vi "UHR-Fleezers Control (fpga) - Lorentz 1.vi"() -> ()   [LabVIEW 2014]
doc: "UHR-Fleezers Instrument Control Code (fpga)"
uses:
  <vilib>/Platform/TimedLoop/XDataNode/timing_clust.ctl
  <vilib>/Platform/TimedLoop/XDataNode/nitl_modes.ctl
  <vilib>/Platform/TimedLoop/XDataNode/wakeup.ctl
  <vilib>/rvi/Emulation/niFpgaGetClockAttributes.vi
  <vilib>/rvi/Emulation/niFpgaSctlEmulationGetInTimedLoop.vi
  <vilib>/rvi/Emulation/niFpgaEmulationReportErrorSimple.vi
  <vilib>/rvi/Emulation/niFpgaProcessEmulError.vi
  <vilib>/rvi/eio/common/nirviEmuTemplateMethod_errors.vi
  <vilib>/rvi/interface/RandomDataEmulation/niFpgaRandomDataHandleErrors.vi
  <vilib>/rvi/Emulation/niFpgaCriticalErrorInLSC.vi
  <vilib>/eio/EIONode/EIONode.xnode
  <vilib>/eio/EIOMethodNode/EIOMethodNode.xnode
  <vilib>/rvi/DataTransferAndStorage/Container/XNode/niFpgaContainer.xnode
  <vilib>/rvi/interface/RandomDataEmulation/nirviRandomDataFpgaReadWriteTemplate.vi
  <vilib>/addons/control/pid/fpga.llb/XNode/niFpgaPID.xnode
  <vilib>/Platform/TimedLoop/XDataNode/XDataNode.xnode
  <vilib>/Platform/TimedLoop/XDataNode/XDNodeRunTimeDep.lvlib
panel:
  in  "Tab Control":T1(tab)=enum."MCL trap control"
  in  "Set 3":bool
  in  "Set 2":bool=TRUE
  in  "Set 1":bool=TRUE
  in  "Trap Pos to FIFO":bool
  in  "N of AI1 Int Acq Sets":i16=2 min=1 max=3 step=1
  out "AI Late Counter":u8
  in  "ai count":u16=400
  in  "+ phase":bool
  in  "Phase count adjustment":i16
  out "Relative phase":i16
  in  "AI to FIFO":bool
  out "BD1 Frequency Out 1":u64
  out "BD1 Frequency Out 2":u64
  out "Trap Pos FIFO Timeout":u16
  out "Trap AI FIFO Timeout":u16
  in  "Trap FIFO Set Timeout":i32
  in  "Tab Control 2":T2(tab)
  in  "FB output range":cluster{"output low":i16, "output high":i16}={"output low"=0, "output high"=3000}
  in  "FB Gains":T3={"proportional gain (Kc)"=10, "integral gain (Kc*Ts/Ti)"=5, "derivative gain (Kc*Td/Ts)"=0}
  in  "RD":bool
  in  "Swap F1 and F2":bool
  in  "Cont. Scan":bool
  in  "Abort scan":bool
  in  "Cycles per step":u64
  in  "Scan BD":bool
  in  "Number of scans":u16
  in  "Scan steps":u64
  in  "Scan freq.  increment":i64
  out "Scanning":bool
  in  "Start scan":bool
  in  "OSK Bd 1":bool
  in  "Reset Bd 1":bool
  in  "PMODE":bool
  in  "Direct RF Box \nCommunication":bool
  in  "Data BD 2":u8 format="%08b"
  in  "Data BD 1":u8 format="%08b"
  in  "Address":u8 format="%02x"
  in  "Update Data":bool
  in  "FPGA Controls\n RF Box":bool
  in  "Number Interlace Cycles":u8=2 min=1 max=3
  in  "Interlace Off Parameters":u8=1 min=1 max=3
  in  "Interlace ON/OFF":bool
  out "DIO Relative phase":i16
  in  "Phase count adjustment (DIO)":i16
  in  "+ phase (DIO)":bool
  out "DIO Late Counter":u8
  in  "DIO count 1 (ticks)":u16=400
  in  "DIO count 2 (ticks)":u16=400
  in  "DIO count 3 (ticks)":u16=400
  out "AI2 Y Sum Set 2":i16
  out "AI2 Y Sum Set 1":i16
  in  "FB Setpoint Set 1":i16 min=0 step=1
  in  "FB Reset Set 1":bool
  in  "FB On/Off Set 1":bool
  in  "FB Reset Set 2":bool
  in  "FB On/Off Set 2":bool
  in  "FB Setpoint Set 2":i16 min=0 step=1
  out "Scan I":u64
  in  "Amp switch delay":u8=5
  in  "BD 2 Amplitude 1":u16
  in  "BD 1 Amplitude 1":u16
  in  "BD 2 Frequency 1":u64
  in  "BD 1 Frequency 1":u64
  in  "BD 2 Amplitude 2":u16
  in  "BD 1 Amplitude 2":u16
  in  "BD 2 Frequency 2":u64
  in  "BD 1 Frequency 2":u64
  in  "BD 2 Amplitude 3":u16
  in  "BD 1 Amplitude 3":u16
  in  "BD 2 Frequency 3":u64
  in  "BD 1 Frequency 3":u64
  in  "BD 1 Delay (ticks)":u8
  in  "BD 2 Delay (Ticks)":u8 caption="Count(Ticks)"
  in  "Next trap write delay (ticks)":u8 caption="Count(Ticks)"
  out "Piezo X out":u16
  out "Piezo Y out":u16
  in  "Piezo Trap ON/Off (AO3)":u16
  in  "Piezo Trap X (AO5)":u16
  in  "Piezo Trap Y (AO4)":u16
  in  "Trap pos. FB Range":T4={"FB2 output low"=-1.0, "FB2 output high"=0.999969482421875}
  in  "FB Min frequency":u64
  in  "FB Max Frequency":u64
  in  "Dynamic Force FB (Ronen)":bool
  in  "Negate Diff?":bool
  in  "Diff FB Measurement?":bool
  in  "FB Trig Integrate":u32=1
  out "TTrig?":bool
  in  "TTrig Negate Pos":bool=TRUE
  out "Trap Pos FB Int Signal":fxp<+/-,24,9> format="%.18g"
  out "Trap Pos FB Int-Norm Signal":fxp<+/-,16,1> format="%.16g"
  in  "FPGA TTrig Thresh":i64
  in  "FPGA Trap Trig":bool
  out "Trap Pos FB Action":i64
  in  "Trap Pos. FB Offset Factor":i64
  in  "Trap Pos. FB Mult Factor":i64=2
  in  "Trap Pos. FB Reset":bool
  in  "Trap Pos FB Monitor T1 or T2":bool
  in  "AI1 X Scale":u16
  in  "Trap Pos FB Int Count":u16=100
  in  "Trap Pos FB Negate Action":bool
  out "AI1 X Set 2":fxp<+/-,16,1>
  out "AI1 X Set 1":fxp<+/-,16,1>
  in  "Trap Pos. FB SP":fxp<+/-,16,1>
  in  "Force feedback":bool
  out "TTrig Sig":i64
  out "TTrig Fin Thresh":i64
  in  "B factor":fxp<+/-,32,16>
  in  "Trap Pos. FB Gains":T5={"proportional gain (Kc)"=0.999969482421875, "integral gain (Kc*Ts/Ti)"=0.999969482421875, "derivative gain (Kc*Td/Ts)"=0.0}
  in  "1D or 2D Scan?":bool
  in  "Abort scan (MCL)":bool
  in  "MCL Scan Axis":bool
  in  "Cont. Scan (MCL)":bool
  out "Scan I (MCL)":u64
  in  "Number of scans (MCL)":u16
  out "Scanning MCL":bool
  in  "Scan steps (MCL)":u64
  in  "Cycles per step (MCL)":u64
  in  "Scan freq.  increment (MCL)":i16
  in  "Start scan (MCL)":bool
  in  "AO2":i16
  in  "AO1":i16
  out "MCL Late Counter":u8
  in  "MCL count":u32=800
  out "MCL Relative Phase":i16
  in  "Phase count adjustment (MCL)":i16
  in  "+ phase (MCL)":bool
  out "APD2 int gate":bool
  out "APD3 out state":bool
  in  "APD Gate Operating Mode":u8 max=2 step=1
  in  "Invert APD Gate":bool
  in  "APD Gate OFF Count":u16=100
  in  "APD Gate ON Count":u16=300
  out "APD 1 Gate Late Counter":u8
  out "APD 1 Gate Relative Phase":i16
  in  "Phase count adjustment (APD 1 Gate)":i16
  in  "+ phase (APD 1 Gate)":bool
  out "APD 2 Counts 0":u32
  out "APD 2 Counts 1":u32
  out "APD 1 Counts 0":u32
  out "APD 1 Counts 1":u32
  out "APD1 out state":bool
  in  "APD AO scale factor":i16=1
  in  "APD to FIFO":bool
  in  "APD Acq Rate Count":u32=20000000
  out "APD Acq Late Counter":u8
  out "APD Acq Relative Phase":i16
  in  "Phase Count Adjustment (APD Acq)":i16
  in  "+ phase (APD Acq)":bool
  in  "Phase count adjustment (APD 2 Gate)":i16
  out "APD 2 Gate Late Counter":u8
  out "APD 2 Gate Relative Phase":i16
  in  "+ phase (APD 2 Gate)":bool
  out "APD2 out state":bool
  out "APD 3 Counts 0":u32
  out "APD 3 Counts 1":u32
  out "APD 3 Gate Late Counter":u8
  in  "Phase count adjustment (APD 3 Gate)":i16
  out "APD 3 Gate Relative Phase":i16
  in  "+ phase (APD 3 Gate)":bool
  out "APD1 int gate":bool
  out "APD3 int gate":bool
  in  "D3":i16
  in  "I3":i16=5
  in  "P3":i16=10
  in  "Green Filter Flipper":bool
  in  "Green FB Count":u16=1200
  out "Green Late Counter":u8
  out "Green FB Relative Phase":i16
  in  "Phase count adjustment (Green FB)":i16=10
  in  "+ phase (Green FB)":bool
  out "Green FB Sum":i16
  in  "Green int current ON count adj":u16=150
  in  "Current Out":u16=30000
  in  "Green FB On/Off":bool
  in  "Green FB Setpoint":i16=250 min=0 step=1
  in  "Green FB Reset":bool
  in  "Operating Mode 2":u8=2 max=2 step=1
  in  "Invert GI 2":bool
  in  "Green interlace OFF count 2":u16=900
  in  "Green interlace ON count 2":u16=300
  out "GI Late Counter 2":u8
  out "GI Relative phase 2":i16
  in  "Phase count adjustment (GI) 2":i16=20
  in  "+ phase (GI) 2":bool
  in  "Green interlace OFF count":u16=100
  out "GI Relative phase":i16
  in  "Phase count adjustment (GI)":i16
  in  "+ phase (GI)":bool
  in  "Green interlace ON count":u16=300
  out "GI Late Counter":u8
  in  "Invert GI":bool
  in  "Operating Mode":u8 max=2 step=1
  in  "+ phase (RI)":bool
  out "RI Relative phase":i16
  out "RI Late Counter":u8
  in  "Red interlace ON count":u16=300
  in  "Red interlace OFF count":u16=100
  in  "Invert RI":bool
  in  "Red Laser Operating Mode":u8 max=2 step=1
  in  "Phase count adjustment (RI)":i16
  out "Red FB Intensity":i16
  in  "RI Current Out":u16=30000
  in  "Red FB On/Off":bool
  in  "D4":i16
  in  "I4":i16=5
  in  "P4":i16=10
  in  "Red FB Setpoint":i16=250 min=0 step=1
  in  "Red FB Reset":bool
  in  "RI Operating Mode 2":u8=2 max=2 step=1
  in  "Invert RI 2":bool
  in  "Phase count adjustment (BI AO)":i16=20
  in  "Blue current ON count adj (AO)":u16=150
  in  "BI Current Out":i16=30000
  in  "Blue FB On/Off":bool
  in  "D5":i16
  in  "I5":i16=5
  in  "P5":i16=10
  in  "Blue FB Setpoint":i16=250 min=0 step=1
  in  "Blue FB Reset":bool
  in  "BI Operating Mode (AO)":u8=2 max=2 step=1
  in  "Invert BI (AO)":bool
  in  "Blue OFF count (AO)":u16=900
  in  "Blue ON count (AO)":u16=300
  out "BI Late Counter (AO)":u8
  out "BI Relative phase (AO)":i16
  in  "+ phase (BI AO)":bool
  in  "Phase count adjustment (BI D)":i16
  in  "Blue Laser Operating Mode (D)":u8 max=2 step=1
  in  "Invert BI (D)":bool
  in  "Blue interlace OFF count (D)":u16=100
  in  "Blue interlace ON count (D)":u16=300
  out "Blue Late Counter (D)":u8
  out "BI Relative phase (D)":i16
  in  "+ phase (BI D)":bool
  out "Blue Intensity":i16
  # "Only one of these can be on\nat a time:"
  # "Raster Scan AOD"
  # "1 (X)"
  # "2 (Y)"
  # "IR Intensity Feedback (RF BD 1)"
  # "False is usual, True is external loop method"
  # "Parameters if using the external RF switching loop"
  # "Parameters if using the usual internal RF switching method"
  # "FB Triggering Excitation Laser"
  # "Trap Pos. FB Gains"
  # "Trap Pos. FB Range"
  # "AO1 (Y)"
  # "2D"
  # "1D"
  # "AO2 (X)"
  # "APD AO for aligning"
  # "Detection Loop"
  # "Green fluorescent laser digital gate interlacing loop"
  # "0 Forced ON\n1 Forced OFF\n2 Interlacing"
  # "Green FB Gains"
  # "Red fluorescent laser digital gate interlacing loop"
  # "Detection Loop"
  # "0 Forced ON\n1 Forced OFF\n2 Interlacing"
  # "Analog/FB Control Loop\n(Disabled)"
  # "Digital Control Loop"
  # "Blue laser intensity reading"
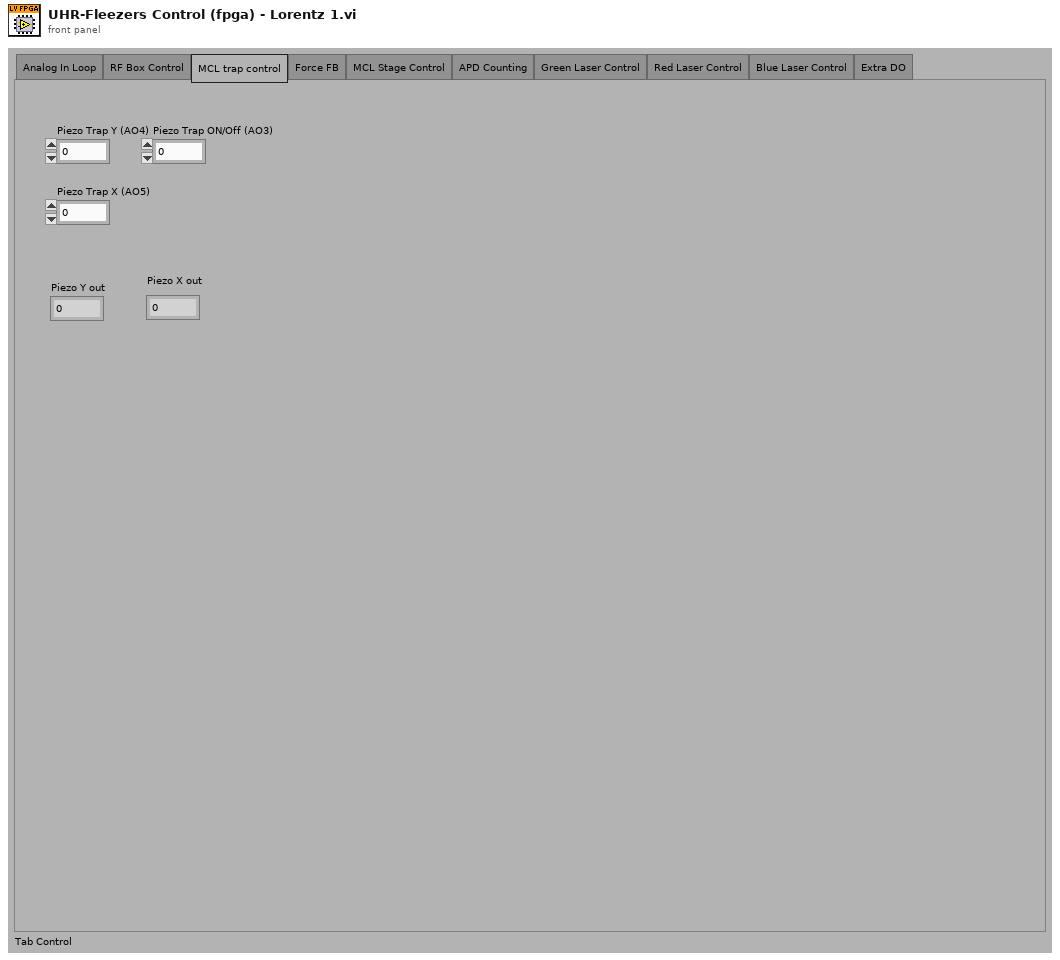
[diagram p1: front panel]
types:
  T1 = enum32{"Analog In Loop", "RF Box Control", "MCL trap control", "Force FB", "MCL Stage Control", "APD Counting", "Green Laser Control", "Red Laser Control", "Blue Laser Control", "Extra DO"}
  T2 = enum32{"Controls", "Interlacing Frequency and Amplitude Values", "Oscillate trap from memory"}
  T3 = cluster{"proportional gain (Kc)":i16, "integral gain (Kc*Ts/Ti)":i16, "derivative gain (Kc*Td/Ts)":i16}
  T4 = cluster{"FB2 output low":fxp<+/-,16,1>, "FB2 output high":fxp<+/-,16,1>}
  T5 = cluster{"proportional gain (Kc)":fxp<+/-,16,1>, "integral gain (Kc*Ts/Ti)":fxp<+/-,16,1>, "derivative gain (Kc*Td/Ts)":fxp<+/-,16,1>}
  T6 = typedef "XDNodeRunTimeDep.lvlib/timing_clust.ctl" = cluster{"Expected End [f-1]":u64, "Actual End [f-1]":u64, "Finished Late? [f-1]":bool, "Expected End [i-1]":u64, "Actual End [i-1]":u64, "Finished Late? [i-1]":bool, "Expected Start [i]":u64, "Actual Start [i]":u64, "Expected Start [f]":u64, "Actual Start [f]":u64, "Source Name":string, "Structure Name":string, "Period":i64, "Deadline":i64, "Offset":i64, "Start":i64, "Priority":i32, "Timeout":i32, "Mode":T7, "Wakeup Reason":T8, "Error":errorcluster, "Source Type":string, "Secondary Source Type":string, "Global End Time":u64, "Global Start Time":u64, "Frame Duration":u64, "Iteration Duration":u64, "Assigned CPU":i32, "I/O Scan Engine Mode":u32}
  T7 = typedef "XDNodeRunTimeDep.lvlib/nitl_modes.ctl" = enum32{"No Change", "Process missed periods, maintain original phase", "Discard missed periods, maintain original phase", "Process missed periods, ignore original phase", "Discard missed periods, ignore original phase"}
  T8 = typedef "XDNodeRunTimeDep.lvlib/wakeup.ctl" = enum32{"Normal", "Aborted", "Asynchronous wakeup", "Timing source error", "Timed loop error", "Timeout"}
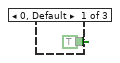
[diagram p2: hidden frame]
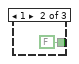
[diagram p3: hidden frame]
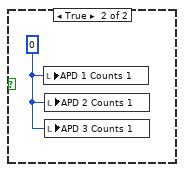
[diagram p5: hidden frame]
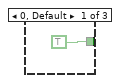
[diagram p7: hidden frame]
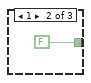
[diagram p8: hidden frame]
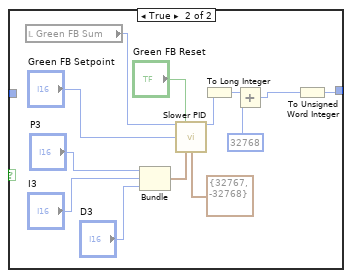
[diagram p11: hidden frame]
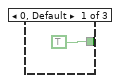
[diagram p12: hidden frame]
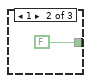
[diagram p13: hidden frame]
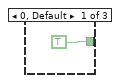
[diagram p14: hidden frame]
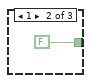
[diagram p15: hidden frame]
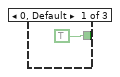
[diagram p17: hidden frame]
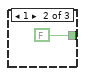
[diagram p18: hidden frame]
diagram:
  w1 = i16 0
  w7 = FALSE
  w5 = FALSE
  # "Control of MCL trap"
  # "timing array current index"
  # "timing array"
  # "timing counter (phase adjusted here)"
  # "late counter"
  n1 = flat-sequence "FPGA initialization to do before running any of the loops" {
    tunnel: [u16 0 ("DIO count 3 (ticks)")] -> w3
    tunnel: [w15] -> _
    frame #0 {
      w14 = FALSE ("Enable")
      # "BD 2 (Y)"
      # "BD 1 (X)"
      # "Start up expansion chassis early\nto avoid delays later"
      # "This pin controls udclk on the RF boards.\nWhen initially configuring the boards, this pin needs to be\nconfigured as a high impedance input.  Later it will be switched\nto an output."
      # "Initial setting of DIO data and \naddress to low (before reset).  \nThis needs to happen before the other\ncontrol method loops execute."
      n2 = xnode "FPGA I/O Node"("Chassis2/Mod1/AO0"=u16 0 ("Chassis2/Mod4/AO0")) -> ("Chassis2/Mod2/AI0"=w15:i16)  [unwired: 2 in, 2 out]
      n3 = xnode "FPGA I/O Method Node"("Enable"=w14) -> ()  [unwired: 1 in, 1 out]
      n4 = xnode "FPGA I/O Method Node"("Enable"=w14) -> ()  [unwired: 1 in, 1 out]
      n5 = xnode "FPGA I/O Node"("Connector1/DIO0"=FALSE, "Connector1/DIO1"=FALSE, "Connector1/DIO2"=FALSE, "Connector1/DIO3"=FALSE, "Connector1/DIO4"=FALSE, "Connector1/DIO5"=FALSE, "Connector1/DIO6"=FALSE, "Connector1/DIO7"=FALSE, "Connector1/DIO8"=FALSE, "Connector1/DIO9"=FALSE, "Connector1/DIO10"=FALSE, "Connector1/DIO11"=FALSE, "Connector1/DIO12"=FALSE, "Connector1/DIO13"=FALSE, "Connector1/DIO15"=FALSE, "Connector1/DIO20"=FALSE, "Connector1/DIO21"=FALSE, "Connector1/DIO22"=FALSE, "Connector1/DIO23"=FALSE, "Connector1/DIO24"=FALSE, "Connector1/DIO25"=FALSE, "Connector1/DIO26"=FALSE, "Connector1/DIO27"=FALSE, "Connector1/DIO14"=FALSE) -> ()  [unwired: 24 in, 24 out]
    }
  }
  n6 = local read "AO1"() -> (w12:i16)
  n7 = local read "AO2"() -> (w11:i16)
  n8 = node-c288() -> (w10:T6)  [unwired: 1 in]
  n9 = To Unsigned Long Integer(number=w3) -> (unsigned 32bit integer=w8:u32)
  n10 = timed-loop "RF box board DIO control: control bits" {
    timing: w10 -> [_]
    timing-out: [_] -> w9
    tunnel: [w44] -> _
    tunnel: w3 -> [w44]
    stop <- FALSE stop-if-true
    n11 = xnode "FPGA I/O Node"("Connector1/DIO16"="RD", "Connector1/DIO17"="PMODE", "Connector1/DIO18"="OSK Bd 1", "Connector1/DIO19"="Reset Bd 1", "Connector0/DIO3"="Green Filter Flipper") -> ()  [unwired: 5 in, 5 out]
  }
  n12 = while "RF box board DIO control: parallel communication" {
    shift-right: [w65] -> _
    shift-left: w3 -> [w64]
    shift-right: [w63] -> _
    shift-left: FALSE ("Swap F1 and F2") -> [w62]
    shift-right: [w57] -> _
    shift-left: u64 0 -> [w58]
    shift-right: [w54] -> _
    shift-left: i16 0 -> [w55]
    shift-right: [w53] -> _
    shift-left: w1 -> [w56]
    shift-right: [w52] -> _
    shift-left: w1 -> [w51]
    stop <- FALSE stop-if-true
    n13 = flat-sequence {
      tunnel: w62 -> [w69]
      tunnel: w64 -> [w67]
      tunnel: [w69] -> w61
      tunnel: [w68] -> w60
      tunnel: [w67] -> w59
      tunnel: [w83] -> w65
      tunnel: [w82] -> w63
      tunnel: w61 -> [w81]
      tunnel: w60 -> [w79]
      tunnel: w59 -> [w78]
      tunnel: w58 -> [w77]
      tunnel: [w76] -> w57
      tunnel: w56 -> [w75]
      tunnel: w55 -> [w74]
      tunnel: [w73] -> w54
      tunnel: [w72] -> w53
      tunnel: [w71] -> w52
      tunnel: w51 -> [w70]
      frame #0 {
        n14 = call "Loop Timer"("Count(Ticks)"=w67) -> ("Tick Count(Ticks)"=w68:u16)
      }
      frame #1 {
        n15 = flat-sequence {
          tunnel: ["FPGA Controls\n RF Box"] -> w80
          tunnel: w81 -> [w87]
          tunnel: w75 -> [w86]
          tunnel: w74 -> [w85]
          tunnel: w70 -> [w84]
          tunnel: [w148] -> w83
          tunnel: [w161] -> w82
          tunnel: w80 -> [w160]
          tunnel: w79 -> [w154]
          tunnel: w78 -> [w151]
          tunnel: w77 -> [w126]
          tunnel: [w125] -> w76
          tunnel: ["Piezo Trap Y (AO4)"] -> w73
          tunnel: ["Piezo Trap X (AO5)"] -> w72
          tunnel: ["Piezo Trap ON/Off (AO3)"] -> w71
          frame #0 {
            n16 = case shown="True" "FPGA Controls\n RF Box" {
              tunnel: w87 -> [_ w92]
              tunnel: w86 -> [_ w91]
              tunnel: w85 -> [_ w90]
              tunnel: w84 -> [_ w89]
              frame False {
              }
              frame True {
                n17 = flat-sequence {
                  tunnel: w92 -> [w102]
                  tunnel: w91 -> [w119]
                  tunnel: w90 -> [w118]
                  tunnel: w89 -> [w117]
                  frame #0 {
                    n18 = First Call?() -> (First Call?: T/F=w93:bool)
                    n19 = case shown="True" w93 {
                      frame False {
                      }
                      frame True {
                        # "BD 2"
                        # "BD 1"
                        # "If first time data updated, be sure to set WR high and UDCLK low\nbefore setting data and address bits."
                        n20 = xnode "FPGA I/O Method Node"("Enable"=TRUE) -> ("FPGA I/O Out"=w95:refnum<k21>)  [unwired: 1 in]
                        n21 = xnode "FPGA I/O Method Node"("Enable"=TRUE) -> ("FPGA I/O Out"=w98:refnum<k21>)  [unwired: 1 in]
                        n22 = xnode "FPGA I/O Node"("Connector1/DIO15"=TRUE) -> ()  [unwired: 1 in, 1 out]
                        n23 = xnode "FPGA I/O Node"("I/O Item"=FALSE ("Connector1/DIO30"), "FPGA I/O In"=w95) -> ()  [unwired: 1 out]
                        n24 = xnode "FPGA I/O Node"("I/O Item"=FALSE ("Connector1/DIO30"), "FPGA I/O In"=w98) -> ()  [unwired: 1 out]
                      }
                    }
                  }
                  frame #1 {
                    n25 = case shown="False" FALSE {
                      tunnel: w102 -> [w104 _]
                      frame False {
                        # "Usual operation"
                        n26 = disable-structure shown="Disabled" {
                          disable-tunnel: w104 -> [w106 _]
                          disable-tunnel: "Amp switch delay" -> [w105 _]
                          frame Disabled {
                            n27 = flat-sequence "BD 2 (Y)" {
                              tunnel: w106 -> [w108]
                              tunnel: w105 -> [w109]
                              frame #0 {
                                n28 = call "Wait7"("Count(Ticks)"="BD 2 Delay (Ticks)") -> ()  [unwired: 1 out]
                              }
                              frame #1 {
                                # "switch frequency"
                                n29 = xnode "FPGA I/O Node"("Connector1/DIO37"=w108) -> ()  [unwired: 1 in, 1 out]
                              }
                              frame #2 {
                                # "~5 ticks is usual"
                                n30 = call "Wait5"("Count(Ticks)"=w109) -> ()  [unwired: 1 out]
                              }
                              frame #3 {
                                # "this switches amplitude"
                                # "switch amplitude"
                                # "send udclk high"
                                n31 = xnode "FPGA I/O Node"("Connector1/DIO29"=TRUE ("Connector1/DIO15")) -> ()  [unwired: 1 in, 1 out]
                              }
                              frame #4 {
                                # "reset to be ready for next\ncycle"
                                # "send udclk low"
                                n32 = xnode "FPGA I/O Node"("Connector1/DIO29"=FALSE ("Connector1/DIO15")) -> ()  [unwired: 1 in, 1 out]
                              }
                            }
                          }
                          frame Enabled {
                          }
                        }
                        n33 = flat-sequence "BD 1 (X)" {
                          tunnel: w104 -> [w113]
                          tunnel: "Amp switch delay" -> [w114]
                          frame #0 {
                            n34 = call "Wait6"("Count(Ticks)"="BD 1 Delay (ticks)") -> ()  [unwired: 1 out]
                          }
                          frame #1 {
                            # "switch frequency"
                            n35 = xnode "FPGA I/O Node"("Connector1/DIO36"=w113) -> ()  [unwired: 1 in, 1 out]
                          }
                          frame #2 {
                            # "~5 ticks is usual"
                            n36 = call "Wait4"("Count(Ticks)"=w114) -> ()  [unwired: 1 out]
                          }
                          frame #3 {
                            # "this switches amplitude"
                            # "switch amplitude"
                            # "send udclk high"
                            n37 = xnode "FPGA I/O Node"("Connector1/DIO30"=TRUE ("Connector1/DIO15")) -> ()  [unwired: 1 in, 1 out]
                          }
                          frame #4 {
                            # "reset to be ready for next\ncycle"
                            # "send udclk low"
                            n38 = xnode "FPGA I/O Node"("Connector1/DIO30"=FALSE ("Connector1/DIO15")) -> ()  [unwired: 1 in, 1 out]
                          }
                        }
                      }
                      frame True {
                        # "Operation when you need a long delay for either X or Y to synchonize AOD light out phase (> ~100 ticks)."
                        # "Trigger the external loop by sending the boolean FSK value through a FIFO"
                      }
                    }
                  }
                  frame #2 {
                    n39 = xnode "FPGA I/O Node"("Connector0/AO4"=w118, "Connector0/AO5"=w119, "Connector0/AO3"=w117) -> ()  [unwired: 3 in, 3 out]
                  }
                }
              }
            }
          }
          frame #1 {
            # "This is the prior cycle's on time"
            # "increment timing\nindex, reset to 0 if \nend of matrix"
            # "Reset to begginning (1) when number of cycles reached."
            # "timing index"
            # "build byte stacks for writing data\n(must correspond to addresses array constant)"
            # "Timing housekeeping"
            # "Adjust phase if late\n(maintains constant phase relationship between cycles)"
            n40 = feedback #1(u8 0 ("t")) -> (w157:u8)
            n41 = Increment(x=w157) -> (x+1=w200:u8)
            n42 = Increment(x="Number Interlace Cycles") -> (x+1=w195:u8)
            n43 = Equal?(x=w200, y=w195) -> (x = y?=w202:bool)
            n44 = Select(t=u8 1, s=w202, f=w200) -> (s? t:f=w156:u8)
            n45 = feedback-in #1(w156) -> ()
            n46 = Increment(x=w156) -> (x+1=w197:u8)
            n47 = Equal?(x=w197, y=w195) -> (x = y?=w198:bool)
            n48 = Select(t=u8 1, s=w198, f=w197) -> (s? t:f=w194:u8)
            n49 = Select(t=w194, s="Interlace ON/OFF", f="Interlace Off Parameters") -> (s? t:f=w127:u8)
            n50 = case shown="1, Default" w127 {
              tunnel: [w246 w455 "BD 1 Frequency 3"] -> w190
              tunnel: [w289 "BD 2 Frequency 2" "BD 2 Frequency 3"] -> w179
              tunnel: ["BD 2 Amplitude 1" "BD 2 Amplitude 2" "BD 2 Amplitude 3"] -> w136
              tunnel: [w255 w453 "BD 1 Amplitude 3"] -> w139
              tunnel: "FB output range" -> [w259 w450 _]
              tunnel: w126 -> [w254 w452 w468]
              tunnel: [w246 w452 w468] -> w125
              tunnel: "FB Gains" -> [w241 w451 _]
              frame 1, Default {
                w273 = fxp<+/-,24,9> 0.0 ("AI1 X Set 2")
                w267 = u16 0
                w285 = u64 0 ("f")
                # "Added by Ronen -\nUpper and Lower \nLimits for the FB \ngenerated frequency\nto avoid losing bead \nwhen tether breaks"
                # "Changed by Ronen - correction \nby PID is now implemented not on \nthe Base BD1 frequency but on the last\nfrequency sent."
                # "BD1 Amp 1"
                # "This signal integration happens no matter what\nso that correct setpoints can be chosen before \nturning on the FB."
                # "Trap 1"
                n51 = local read "AI1 X Set 2"() -> (w249:fxp<+/-,16,1>)
                n52 = local read "AI1 X Set 1"() -> (w270:fxp<+/-,16,1>)
                n53 = local read "Scanning"() -> (w290:bool)
                n54 = Multiply(x=w249, y="B factor") -> (x*y=w247:fxp<+/-,48,17>)
                n55 = Or(x=w290, y="Start scan") -> (x .or. y?=w283:bool)
                n56 = case shown="True" "Diff FB Measurement?" {
                  tunnel: w247 -> [w308 w317]
                  tunnel: w270 -> [w307 w318]
                  tunnel: [w305 w309] -> w271
                  frame False {
                    n57 = Select(t=w307, s="Trap Pos FB Monitor T1 or T2", f=w308) -> (s? t:f=w305:fxp<+/-,48,17>)
                  }
                  frame True {
                    n58 = Subtract(x=w318, y=w317) -> (x-y=w310:fxp<+/-,48,17>)
                    n59 = Not(x="Negate Diff?") -> (.not. x?=w316:bool)
                    n60 = Boolean To (0,1)(Boolean="Negate Diff?") -> (0, 1=w314:i16)
                    n61 = Boolean To (0,1)(Boolean=w316) -> (0, 1=w315:i16)
                    n62 = Negate(x=w314) -> (-x=w313:i16)
                    n63 = Add(x=w313, y=w315) -> (x+y=w311:i16)
                    n64 = Multiply(x=w311, y=w310) -> (x*y=w309:fxp<+/-,63,32>)
                  }
                }
                n65 = Not(x="Abort scan") -> (.not. x?=w281:bool)
                n66 = And(x=w281, y=w283) -> (x .and. y?=w280:bool)
                n67 = case "For raster scanning" shown="True" w280 {
                  tunnel: [u64 0 w440] -> w286
                  tunnel: "Start scan" -> [_ w425]
                  frame False {
                    n68 = local write "Scanning"(FALSE ("scanning")) -> ()
                  }
                  frame True {
                    w409 = i64 0
                    w408 = u64 0
                    # "scan incr."
                    # "freq. incr. mult."
                    # "count steps"
                    # "count number of cycles"
                    n69 = feedback #2(w408) -> (w437:u64)
                    n70 = Select(t=w408, s=w425, f=w437) -> (s? t:f=w439:u64)
                    n71 = Increment(x=w439) -> (x+1=w436:u64)
                    n72 = Greater?(x="Cycles per step", y=w436) -> (0:w418:bool)
                    n73 = Select(t=w436, s=w418, f=w408) -> (s? t:f=w435:u64)
                    n74 = feedback-in #2(w435) -> ()
                    n75 = feedback #3(w408) -> (w434:u64)
                    n76 = Select(t=w408, s=w425, f=w434) -> (s? t:f=w429:u64)
                    n77 = Increment(x=w429) -> (x+1=w433:u64)
                    n78 = Add(x="Scan steps", y="Scan steps") -> (x+y=w432:u64)
                    n79 = Select(t=w429, s=w418, f=w433) -> (s? t:f=w413:u64)
                    n80 = Greater?(x=w432, y=w413) -> (0:w412:bool)
                    n81 = Select(t=w413, s=w412, f=w408) -> (s? t:f=w430:u64)
                    n82 = feedback-in #3(w430) -> ()
                    n83 = Equal?(x="Scan steps", y=w413) -> (x = y?=w417:bool)
                    n84 = Greater?(x="Scan steps", y=w429) -> (0:w428:bool)
                    n85 = feedback #4(w409) -> (w431:i64)
                    n86 = Select(t=w409, s=w425, f=w431) -> (s? t:f=w415:i64)
                    n87 = Increment(x=w415) -> (x+1=w427:i64)
                    n88 = Decrement(x=w415) -> (x-1=w426:i64)
                    n89 = Select(t=w427, s=w428, f=w426) -> (s? t:f=w416:i64)
                    n90 = Select(t=w415, s=w417, f=w416) -> (s? t:f=w414:i64)
                    n91 = Select(t=w415, s=w418, f=w414) -> (s? t:f=w410:i64)
                    n92 = Select(t=w410, s=w412, f=w409) -> (s? t:f=w411:i64)
                    n93 = feedback-in #4(w411) -> ()
                    n94 = feedback #5(w408) -> (w424:u64)
                    n95 = Select(t=w408, s=w425, f=w424) -> (s? t:f=w420:u64)
                    n96 = Increment(x=w420) -> (x+1=w421:u64)
                    n97 = Select(t=w420, s=w412, f=w421) -> (s? t:f=w419:u64)
                    n98 = Greater?(x="Number of scans", y=w419) -> (0:w405:bool)
                    n99 = Multiply(x="Scan freq.  increment", y=w415) -> (x*y=w440:i64)
                    n100 = Select(t=TRUE, s="Cont. Scan", f=w405) -> (s? t:f=w404:bool)
                    "Scanning" <- w404
                    n101 = Select(t=w419, s=w404, f=w408) -> (s? t:f=w422:u64)
                    n102 = feedback-in #5(w422) -> ()
                    n103 = Increment(x=w419) -> (x+1=→"Scan I":u64)
                  }
                }
                n104 = feedback #6(w267) -> (w266:u16)
                n105 = Increment(x=w266) -> (x+1=w268:u16)
                n106 = Greater Or Equal?(x=w268, y="Trap Pos FB Int Count") -> (x >= y?=w253:bool)
                n107 = Select(t=w267, s=w253, f=w268) -> (s? t:f=w269:u16)
                n108 = feedback-in #6(w269) -> ()
                n109 = feedback #7(w273) -> (w272:fxp<+/-,24,9>)
                n110 = Add(x=w271, y=w272) -> (x+y=w265:fxp<+/-,24,9>)
                n111 = case "For intensity feedback" shown="True" "FB On/Off Set 1" {
                  tunnel: [w442 w448] -> w255
                  tunnel: w259 -> [_ w449]
                  tunnel: "BD 1 Amplitude 1" -> [w442 _]
                  tunnel: w241 -> [_ w443]
                  frame False {
                  }
                  frame True {
                    n112 = local read "AI2 Y Sum Set 1"() -> (w446:i16)
                    n113 = call "Slower PID.vi"("process variable"=w446, "reset?"="FB Reset Set 1", "setpoint"="FB Setpoint Set 1", "PID gains (x 2^8)"=w443, "output range"=w449) -> ("output"=w444:i16)  [unwired: 10 out]
                    n114 = To Unsigned Word Integer(number=w444) -> (unsigned 16bit integer=w448:u16)
                  }
                }
                n115 = Select(t=w273, s=w253, f=w265) -> (s? t:f=w276:fxp<+/-,24,9>)
                n116 = feedback-in #7(w276) -> ()
                n117 = Divide(x=w265, y="Trap Pos FB Int Count") -> (x/y=w260:fxp<+/-,16,1>)
                n118 = feedback #8(fxp<+/-,24,9> 0.0 ("AI1 X Set 2")) -> (w277:fxp<+/-,24,9>)
                n119 = Select(t=w265, s=w253, f=w277) -> (s? t:f=w278:fxp<+/-,24,9>)
                "Trap Pos FB Int Signal" <- w278
                n120 = feedback-in #8(w278) -> ()
                n121 = feedback #9(fxp<+/-,16,1> 0.0 ("Trap Pos FB Int-Norm Signal")) -> (w262:fxp<+/-,16,1>)
                n122 = Select(t=w260, s=w253, f=w262) -> (s? t:f=w261:fxp<+/-,16,1>)
                "Trap Pos FB Int-Norm Signal" <- w261
                n123 = feedback-in #9(w261) -> ()
                n124 = case "For position feedback" shown="True" "Force feedback" {
                  tunnel: [i64 0 w324] -> w258
                  tunnel: w260 -> [_ w321]
                  tunnel: w253 -> [_ w320]
                  frame False {
                  }
                  frame True {
                    n125 = feedback #10(i64 0) -> (w323:i64)
                    n126 = case shown="True" w320 {
                      tunnel: [w325 w329] -> w324
                      tunnel: w323 -> [w325 _]
                      tunnel: w321 -> [_ w328]
                      frame False {
                      }
                      frame True {
                        n127 = xnode ("PID")("process variable"=w328, "reset?"="Trap Pos. FB Reset", "setpoint"="Trap Pos. FB SP", "PID gains"="Trap Pos. FB Gains", "output range"="Trap pos. FB Range") -> ("output"=w338:fxp<+/-,16,1>)
                        n128 = Negate(x=w338) -> (-x=w337:fxp<+/-,17,2>)
                        n129 = Select(t=w337, s="Trap Pos FB Negate Action", f=w338) -> (s? t:f=w334:fxp<+/-,17,2>)
                        n130 = Scale By Power Of 2(n=u32 15, x=u32 1) -> (x*2^n=w331:u32)
                        n131 = Multiply(x=w334, y=w331) -> (x*y=w330:fxp<+/-,17,17>)
                        n132 = To Quad Integer(1:w330) -> (0:w342:i64)
                        "Trap Pos FB Action" <- w342
                        n133 = Multiply(x=w342, y="Trap Pos. FB Mult Factor") -> (x*y=w340:i64)
                        n134 = Add(x=w340, y="Trap Pos. FB Offset Factor") -> (x+y=w329:i64)
                        n135 = disable-structure shown="Disabled" {
                          disable-tunnel: w329 -> [w349 _]
                          frame Disabled {
                            w353 = u32 0
                            n136 = feedback #11() -> (w350:i64)  [unwired: 1 in]
                            n137 = Add(x=w349, y=w350) -> (x+y=w347:i64)
                            n138 = feedback #12(w353) -> (w355:u32)
                            n139 = Increment(x=w355) -> (x+1=w344:u32)
                            n140 = Greater Or Equal?(x=w344, y="FB Trig Integrate") -> (x >= y?=w345:bool)
                            n141 = Select(t=i64 0, s=w345, f=w347) -> (s? t:f=w351:i64)
                            n142 = feedback-in #11(w351) -> ()
                            n143 = Select(t=w353, s=w345, f=w344) -> (s? t:f=w354:u32)
                            n144 = feedback-in #12(w354) -> ()
                            n145 = And(x=w345, y="FPGA Trap Trig") -> (x .and. y?=w352:bool)
                            n146 = case "Trap FB trigger excitation laser ON" shown="True" w352 {
                              tunnel: w347 -> [_ w359]
                              tunnel: w344 -> [_ w357]
                              frame False {
                              }
                              frame True {
                                n147 = Not(x="TTrig Negate Pos") -> (.not. x?=w366:bool)
                                n148 = Boolean To (0,1)(Boolean="TTrig Negate Pos") -> (0, 1=w364:i16)
                                n149 = Boolean To (0,1)(Boolean=w366) -> (0, 1=w365:i16)
                                n150 = Negate(x=w364) -> (-x=w363:i16)
                                n151 = Add(x=w363, y=w365) -> (x+y=w362:i16)
                                n152 = Multiply(x=w362, y=w359) -> (x*y=w361:i64)
                                "TTrig Sig" <- w361
                                n153 = Multiply(x="FPGA TTrig Thresh", y=w357) -> (x*y=w358:i64)
                                "TTrig Fin Thresh" <- w358
                                n154 = Greater Or Equal?(x=w361, y=w358) -> (x >= y?=w360:bool)
                                n155 = case shown="True" w360 {
                                frame False {
                                }
                                frame True {
                                w369 = TRUE ("Green FB On/Off")
                                w371 = u8 2 ("Operating Mode")
                                n156 = local write "Operating Mode 2"(w371) -> ()
                                n157 = local write "Operating Mode"(w371) -> ()
                                n158 = local write "Green FB On/Off"(w369) -> ()
                                n159 = local write "FPGA Trap Trig"(FALSE ("FPGA Trap Trig")) -> ()
                                "TTrig?" <- w369
                                }
                                }
                              }
                            }
                          }
                          frame Enabled {
                          }
                        }
                      }
                    }
                    n160 = feedback-in #10(w324) -> ()
                  }
                }
                n161 = And(x="Force feedback", y="Dynamic Force FB (Ronen)") -> (x .and. y?=w243:bool)
                n162 = case shown="True" w243 {
                  tunnel: w258 -> [w296 w300]
                  tunnel: [w295 w299] -> w256
                  tunnel: w254 -> [_ w298]
                  tunnel: w253 -> [_ w297]
                  frame False {
                    # "(BD1 Frequency 1)"
                    n163 = Add(x="BD 1 Frequency 1", y=w296) -> (x+y=w295:u64)
                  }
                  frame True {
                    n164 = case shown="True" w297 {
                      tunnel: w300 -> [_ w304]
                      tunnel: [w301 w303] -> w299
                      tunnel: w298 -> [w301 w302]
                      frame False {
                      }
                      frame True {
                        n165 = Add(x=w302, y=w304) -> (x+y=w303:u64)
                      }
                    }
                  }
                }
                n166 = Select(t=w285, s="Scan BD", f=w286) -> (s? t:f=w284:u64)
                n167 = Select(t=w286, s="Scan BD", f=w285) -> (s? t:f=w287:u64)
                n168 = Add(x=w284, y="BD 2 Frequency 1") -> (x+y=w289:u64)
                n169 = Compound Arithmetic op=ADD(i64 0 ("f"), w256, w287) -> (w252:u64)
                n170 = In Range and Coerce(upper limit="FB Max Frequency", x=w252, lower limit="FB Min frequency") -> (coerced(x)=w246:u64)  [unwired: 1 out]
                "BD1 Frequency Out 1" <- w246
              }
              frame 2 {
                # "Trap 2"
                n171 = case shown="True" "FB On/Off Set 2" {
                  tunnel: ["BD 1 Amplitude 2" w463] -> w453
                  tunnel: w450 -> [_ w464]
                  tunnel: w451 -> [_ w461]
                  frame False {
                  }
                  frame True {
                    n172 = local read "AI2 Y Sum Set 2"() -> (w466:i16)
                    n173 = call "Slower PID.vi"("process variable"=w466, "reset?"="FB Reset Set 2", "setpoint"="FB Setpoint Set 2", "PID gains (x 2^8)"=w461, "output range"=w464) -> ("output"=w462:i16)  [unwired: 10 out]
                    n174 = To Unsigned Word Integer(number=w462) -> (unsigned 16bit integer=w463:u16)
                  }
                }
                n175 = Add(x="BD 1 Frequency 2", y=i64 0 ("f")) -> (x+y=w455:u64)
                "BD1 Frequency Out 2" <- w455
              }
              frame 3 {
                # "Fluorescence period"
              }
            }
            n176 = feedback-in #13(w154) -> ()
            n177 = feedback #13(w154) -> (w153:u16)
            n178 = Select(t=w156, s="Interlace ON/OFF", f="Interlace Off Parameters") -> (s? t:f=w193:u8)
            n179 = Subtract(x=w154, y=w153) -> (x-y=w152:u16)
            n180 = Subtract "The error"(x=w152, y=w151) -> (x-y=w129:u16)
            n181 = case shown="1, Default" w193 {
              tunnel: ["DIO count 1 (ticks)" "DIO count 2 (ticks)" "DIO count 3 (ticks)"] -> w150
              frame 1, Default {
              }
              frame 2 {
              }
              frame 3 {
              }
            }
            n182 = Number To Boolean Array(number=w129) -> (Boolean array=w130:bool[])
            n183 = Or Array Elements(Boolean array=w130) -> (logical OR=w128:bool)
            n184 = Boolean To (0,1)(Boolean=w128) -> (0, 1=w135:i16)
            n185 = To Unsigned Byte Integer(number=w135) -> (unsigned 8bit integer=w132:u8)
            n186 = feedback #14(u8 0) -> (w133:u8)
            n187 = Add(x=w132, y=w133) -> (x+y=w131:u8)
            "DIO Late Counter" <- w131
            n188 = feedback-in #14(w131) -> ()
            n189 = Subtract(x=w150, y=w129) -> (x-y=w149:u16)
            n190 = Split Number(x=w190) -> (hi(x)=w189:u32, lo(x)=w188:u32)
            n191 = Split Number(x=w179) -> (hi(x)=w184:u32, lo(x)=w183:u32)
            n192 = Boolean To (0,1)(Boolean="+ phase (DIO)") -> (0, 1=w146:i16)
            n193 = Split Number(x=w189) -> (lo(x)=w187:u16)  [unwired: 1 out]
            n194 = Split Number(x=w188) -> (hi(x)=w186:u16, lo(x)=w185:u16)
            n195 = Split Number(x=w184) -> (lo(x)=w182:u16)  [unwired: 1 out]
            n196 = Split Number(x=w183) -> (hi(x)=w181:u16, lo(x)=w180:u16)
            n197 = Split Number(x=w139) -> (hi(x)=w141:u8, lo(x)=w140:u8)
            n198 = Split Number(x=w136) -> (hi(x)=w138:u8, lo(x)=w137:u8)
            n199 = Split Number(x=w187) -> (hi(x)=w178:u8, lo(x)=w177:u8)
            n200 = Split Number(x=w186) -> (hi(x)=w176:u8, lo(x)=w175:u8)
            n201 = Split Number(x=w182) -> (hi(x)=w171:u8, lo(x)=w170:u8)
            n202 = Split Number(x=w185) -> (hi(x)=w174:u8, lo(x)=w173:u8)
            n203 = Split Number(x=w181) -> (hi(x)=w169:u8, lo(x)=w168:u8)
            n204 = Split Number(x=w180) -> (hi(x)=w167:u8, lo(x)=w166:u8)
            n205 = Multiply(x=w146, y="Phase count adjustment (DIO)") -> (x*y=w142:i16)
            n206 = feedback #15(i16 0) -> (w144:i16)
            n207 = Subtract(x=w144, y=w142) -> (x-y=w143:i16)
            "DIO Relative phase" <- w143
            n208 = feedback-in #15(w143) -> ()
            n209 = Add(x=w149, y=w142) -> (x+y=w148:u16)
            n210 = Build Array "BD 1 A Stack"(w141, w140) -> (w163:u8[])
            n211 = Build Array "BD 2 A Stack"(w138, w137) -> (w162:u8[])
            n212 = Build Array "BD 1 nu Stack"(w178, w177, w176, w175, w174, w173) -> (w172:u8[])
            n213 = Build Array "BD 2 nu Stack"(w171, w170, w169, w168, w167, w166) -> (w165:u8[])
            n214 = case shown="2" w127 {
              tunnel: [w233 w236] -> w161
              tunnel: [u8 10 u8 4] -> w164
              tunnel: "Swap F1 and F2" -> [w234 w236]
              frame 2 {
                # "F2"
                n215 = Not(x=w234) -> (.not. x?=w233:bool)
              }
              frame 1, Default {
                # "low chooses F1"
                # "F1"
              }
            }
            n216 = case "If FPGA is controlling (toggling) RF synth" shown="True" w160 {
              tunnel: w172 -> [_ w209]
              tunnel: w165 -> [_ w208]
              tunnel: w164 -> [_ w207]
              tunnel: w163 -> [_ w206]
              tunnel: w162 -> [_ w205]
              frame False {
              }
              frame True {
                # "Write next amp.\n(wait until beginning of next loop iteration to update)"
                n217 = flat-sequence "Update the next F1 and F2 frequency value (the actual frequency won't change until FSK is switched).\nThen load the next amplitude value into buffer, but don't update it until the next cycle." {
                  tunnel: w208 -> [w211]
                  tunnel: w209 -> [w212]
                  tunnel: [w212] -> w204
                  tunnel: [w211] -> w203
                  tunnel: w207 -> [w213]
                  tunnel: w204 -> [w215]
                  tunnel: w203 -> [w214]
                  tunnel: w206 -> [w226]
                  tunnel: w205 -> [w225]
                  frame #0 {
                    # "To possibly send\nthese writes to very\nend of loop (for x and\ny phase adjust)"
                    n218 = call "Wait8"("Count(Ticks)"="Next trap write delay (ticks)") -> ()  [unwired: 1 out]
                  }
                  frame #1 {
                    n219 = for {
                      tunnel: w215 -> [w221] mode=indexing
                      tunnel: w214 -> [w220] mode=indexing
                      tunnel: w213 -> [w218]
                      i -> [w219]
                      # "Write next freq."
                      n220 = To Unsigned Byte Integer(number=w219) -> (unsigned 8bit integer=w216:u8)
                      n221 = Add(x=w218, y=w216) -> (x+y=w217:u8)
                      n222 = call "write to RF synth bd.vi"("Address Byte"=w217, "BD 2 Byte"=w220, "BD 1 Byte"=w221) -> ()
                    }
                  }
                  frame #2 {
                    w222 = TRUE ("Connector1/DIO15")
                    # "send udclk high\n(BD 1 and 2)"
                    n223 = xnode "FPGA I/O Node"("Connector1/DIO30"=w222, "Connector1/DIO29"=w222) -> ()  [unwired: 2 in, 2 out]
                  }
                  frame #3 {
                    w223 = FALSE ("Connector1/DIO15")
                    n224 = xnode "FPGA I/O Node"("Connector1/DIO30"=w223, "Connector1/DIO29"=w223) -> ()  [unwired: 2 in, 2 out]
                  }
                  frame #4 {
                    n225 = for {
                      tunnel: w226 -> [w232] mode=indexing
                      tunnel: w225 -> [w231] mode=indexing
                      tunnel: u8 33 -> [w229]
                      i -> [w230]
                      n226 = To Unsigned Byte Integer(number=w230) -> (unsigned 8bit integer=w227:u8)
                      n227 = Add(x=w229, y=w227) -> (x+y=w228:u8)
                      n228 = call "write to RF synth bd.vi"("Address Byte"=w228, "BD 2 Byte"=w231, "BD 1 Byte"=w232) -> ()
                    }
                  }
                }
              }
            }
            "Piezo Y out" <- "Piezo Trap Y (AO4)"
            "Piezo X out" <- "Piezo Trap X (AO5)"
          }
        }
      }
    }
  }
  n229 = disable-structure shown="Disabled" {
    disable-tunnel: w3 -> [w473 _]
    frame Disabled {
      n230 = while "Excitation laser intensity feedback measurement (all lasers)" {
        shift-right: [w474] -> _
        shift-left: w473 -> [w479]
        stop <- FALSE stop-if-true
        n231 = flat-sequence {
          tunnel: w479 -> [w481]
          tunnel: [w482] -> w477
          tunnel: [w481] -> w475
          tunnel: [w488] -> w478
          tunnel: w477 -> [w488]
          tunnel: [w487] -> w476
          tunnel: w475 -> [w487]
          tunnel: [w500] -> w474
          tunnel: w478 -> [w511]
          tunnel: w476 -> [w508]
          frame #0 {
            n232 = call "Loop Timer9"("Count(Ticks)"=w481) -> ("Tick Count(Ticks)"=w482:u16)
          }
          frame #1 {
            # "Design note:\n\nAll lasers need to be measured at the same \ntime because the AI expansion module\ncannot independently time the measurements\nwithin our requirements: their is dead time.\n\nThis probably wouldn't be an issue with the built\nin AI on the fpga board itself."
            n233 = xnode "FPGA I/O Node"("Connector1/DIO35"=TRUE) -> ("Chassis2/Mod2/AI2"=→"Blue Intensity":i16, "Chassis2/Mod2/AI1"=→"Red FB Intensity":i16, "Chassis2/Mod2/AI0"=→"Green FB Sum":i16)  [unwired: 4 in, 4 out]
          }
          frame #2 {
            n234 = feedback-in #16(w511) -> ()
            n235 = feedback #16(w511) -> (w510:u16)
            n236 = Subtract(x=w511, y=w510) -> (x-y=w509:u16)
            n237 = xnode "FPGA I/O Node"("Connector1/DIO35"=FALSE) -> ()  [unwired: 1 in, 1 out]
            n238 = Subtract(x=w509, y=w508) -> (x-y=w490:u16)
            n239 = Subtract(x="Green FB Count", y=w490) -> (x-y=w504:u16)
            n240 = Number To Boolean Array(number=w490) -> (Boolean array=w491:bool[])
            n241 = Or Array Elements(Boolean array=w491) -> (logical OR=w489:bool)
            n242 = Boolean To (0,1)(Boolean="+ phase (Green FB)") -> (0, 1=w502:i16)
            n243 = Boolean To (0,1)(Boolean=w489) -> (0, 1=w496:i16)
            n244 = Multiply(x=w502, y="Phase count adjustment (Green FB)") -> (x*y=w497:i16)
            n245 = Add(x=w504, y=w497) -> (x+y=w500:u16)
            n246 = To Unsigned Byte Integer(number=w496) -> (unsigned 8bit integer=w493:u8)
            n247 = feedback #17(i16 0) -> (w499:i16)
            n248 = Subtract(x=w499, y=w497) -> (x-y=w498:i16)
            "Green FB Relative Phase" <- w498
            n249 = feedback-in #17(w498) -> ()
            n250 = feedback #18(u8 0) -> (w494:u8)
            n251 = Add(x=w493, y=w494) -> (x+y=w492:u8)
            "Green Late Counter" <- w492
            n252 = feedback-in #18(w492) -> ()
          }
        }
      }
    }
    frame Enabled {
    }
  }
  n253 = while "RF box board direct communication loop" {
    tunnel: w3 -> [_]
    stop <- FALSE stop-if-true
    n254 = case "Whether to use direct communication method (only use one method at a time)" shown="True" "Direct RF Box \nCommunication" {
      frame False {
      }
      frame True {
        n255 = case shown="True" "Update Data" {
          frame False {
          }
          frame True {
            n256 = flat-sequence {
              frame #0 {
                n257 = First Call?() -> (First Call?: T/F=w515:bool)
                n258 = case shown="True" w515 {
                  frame False {
                  }
                  frame True {
                    # "If first time data updated, be sure to set WR high\nbefore setting data and address bits."
                    n259 = flat-sequence {
                      frame #0 {
                        n260 = xnode "FPGA I/O Node"("Connector1/DIO15"=TRUE) -> ()  [unwired: 1 in, 1 out]
                      }
                      frame #1 {
                        n261 = call "Wait"("Count(Ticks)"=u8 40 ("DO Delay 3 (Ticks)")) -> ()  [unwired: 1 out]
                      }
                    }
                  }
                }
              }
              frame #1 {
                n262 = Number To Boolean Array(number="Address") -> (Boolean array=w564:bool[])
                n263 = Number To Boolean Array(number="Data BD 1") -> (Boolean array=w565:bool[])
                n264 = Number To Boolean Array(number="Data BD 2") -> (Boolean array=w534:bool[])
                n265 = Index Array(array=w565, index=7) -> (element=w549:bool)
                n266 = Index Array(array=w565, index=6) -> (element=w548:bool)
                n267 = Index Array(array=w565, index=5) -> (element=w547:bool)
                n268 = Index Array(array=w565, index=4) -> (element=w546:bool)
                n269 = Index Array(array=w565, index=3) -> (element=w545:bool)
                n270 = Index Array(array=w565, index=2) -> (element=w544:bool)
                n271 = Index Array(array=w565, index=1) -> (element=w543:bool)
                n272 = Index Array(array=w565, index=0) -> (element=w542:bool)
                n273 = Index Array(array=w564, index=5) -> (element=w541:bool)
                n274 = Index Array(array=w564, index=4) -> (element=w540:bool)
                n275 = Index Array(array=w564, index=3) -> (element=w539:bool)
                n276 = Index Array(array=w564, index=2) -> (element=w538:bool)
                n277 = Index Array(array=w564, index=1) -> (element=w537:bool)
                n278 = Index Array(array=w564, index=0) -> (element=w536:bool)
                n279 = Index Array(array=w534, index=7) -> (element=w525:bool)
                n280 = Index Array(array=w534, index=6) -> (element=w524:bool)
                n281 = Index Array(array=w534, index=5) -> (element=w523:bool)
                n282 = Index Array(array=w534, index=4) -> (element=w522:bool)
                n283 = Index Array(array=w534, index=3) -> (element=w521:bool)
                n284 = Index Array(array=w534, index=2) -> (element=w520:bool)
                n285 = Index Array(array=w534, index=1) -> (element=w519:bool)
                n286 = Index Array(array=w534, index=0) -> (element=w518:bool)
                n287 = xnode "FPGA I/O Node"("Connector1/DIO0"=w549, "Connector1/DIO1"=w548, "Connector1/DIO2"=w547, "Connector1/DIO3"=w546, "Connector1/DIO4"=w545, "Connector1/DIO5"=w544, "Connector1/DIO6"=w543, "Connector1/DIO7"=w542, "Connector1/DIO8"=w541, "Connector1/DIO9"=w540, "Connector1/DIO10"=w539, "Connector1/DIO11"=w538, "Connector1/DIO12"=w537, "Connector1/DIO13"=w536, "Connector1/DIO20"=w525, "Connector1/DIO21"=w524, "Connector1/DIO22"=w523, "Connector1/DIO23"=w522, "Connector1/DIO24"=w521, "Connector1/DIO25"=w520, "Connector1/DIO26"=w519, "Connector1/DIO27"=w518) -> ()  [unwired: 22 in, 22 out]
              }
              frame #2 {
                # "wait and then apply write signal"
                n288 = call "Wait2"("Count(Ticks)"=u8 40 ("DO Delay 1 (Ticks)")) -> ()  [unwired: 1 out]
              }
              frame #3 {
                # "sending bit low writes data to board buffer"
                n289 = xnode "FPGA I/O Node"("Connector1/DIO15"=FALSE) -> ()  [unwired: 1 in, 1 out]
              }
              frame #4 {
                # "wait then return write signal"
                n290 = call "Wait3"("Count(Ticks)"=u8 40 ("DO Delay 2 (Ticks)")) -> ()  [unwired: 1 out]
              }
              frame #5 {
                # "sending bit high makes ready to\nwrite more data"
                n291 = xnode "FPGA I/O Node"("Connector1/DIO15"=TRUE) -> ()  [unwired: 1 in, 1 out]
              }
            }
          }
        }
      }
    }
  }
  n292 = disable-structure shown="Disabled" {
    disable-tunnel: w7 -> [w573 _]
    disable-tunnel: w3 -> [w572 _]
    frame Disabled {
      n293 = while "APD 2 Gating" {
        shift-right: [w577] -> _
        shift-left: w572 -> [w582]
        shift-right: [w576] -> _
        shift-left: w573 -> [w574]
        stop <- FALSE stop-if-true
        n294 = flat-sequence {
          tunnel: w582 -> [w585]
          tunnel: [w586] -> w580
          tunnel: [w585] -> w578
          tunnel: [w584] -> w575
          tunnel: w574 -> [w584]
          tunnel: [w589] -> w581
          tunnel: w580 -> [w589]
          tunnel: [w588] -> w579
          tunnel: w578 -> [w588]
          tunnel: w575 -> [w587]
          tunnel: [w611] -> w577
          tunnel: w581 -> [w621]
          tunnel: w579 -> [w619]
          tunnel: [w590] -> w576
          frame #0 {
            n295 = call "Loop Timer8"("Count(Ticks)"=w585) -> ("Tick Count(Ticks)"=w586:u16)
          }
          frame #1 {
            # "Signal maybe then sent through \na transistor before APD"
            n296 = xnode "FPGA I/O Node"("Connector0/DIO8"=w587, "Connector0/DIO9"=w587, "Connector0/DIO10"=w587, "Connector0/DIO11"=w587) -> ()  [unwired: 4 in, 4 out]
            "APD2 int gate" <- w587
          }
          frame #2 {
            n297 = local read "APD Gate ON Count"() -> (w604:u16)
            n298 = local read "APD Gate OFF Count"() -> (w603:u16)
            n299 = feedback #19(TRUE) -> (w616:bool)
            n300 = feedback-in #20(w621) -> ()
            n301 = feedback #20(w621) -> (w605:u16)
            n302 = Not(x=w616) -> (.not. x?=w614:bool)
            n303 = feedback-in #19(w614) -> ()
            n304 = Subtract(x=w621, y=w605) -> (x-y=w620:u16)
            n305 = Select(t=w604, s=w614, f=w603) -> (s? t:f=w618:u16)
            n306 = Subtract(x=w620, y=w619) -> (x-y=w596:u16)
            n307 = Subtract(x=w618, y=w596) -> (x-y=w610:u16)
            n308 = Number To Boolean Array(number=w596) -> (Boolean array=w595:bool[])
            n309 = Or Array Elements(Boolean array=w595) -> (logical OR=w594:bool)
            n310 = Boolean To (0,1)(Boolean="+ phase (APD 2 Gate)") -> (0, 1=w608:i16)
            n311 = Multiply(x=w608, y="Phase count adjustment (APD 2 Gate)") -> (x*y=w606:i16)
            n312 = Boolean To (0,1)(Boolean=w594) -> (0, 1=w601:i16)
            n313 = Add(x=w610, y=w606) -> (x+y=w611:u16)
            n314 = To Unsigned Byte Integer(number=w601) -> (unsigned 8bit integer=w598:u8)
            n315 = feedback #21(i16 0) -> (w613:i16)
            n316 = Subtract(x=w613, y=w606) -> (x-y=w612:i16)
            "APD 2 Gate Relative Phase" <- w612
            n317 = feedback-in #21(w612) -> ()
            n318 = feedback #22(u8 0) -> (w599:u8)
            n319 = Add(x=w598, y=w599) -> (x+y=w597:u8)
            "APD 2 Gate Late Counter" <- w597
            n320 = feedback-in #22(w597) -> ()
            n321 = local read "APD Gate Operating Mode"() -> (w602:u8)
            n322 = case shown="2" w602 {
              tunnel: [TRUE FALSE w624] -> w591
              tunnel: w616 -> [_ _ w624]
              frame 0, Default {
              }
              frame 1 {
              }
              frame 2 {
              }
            }
            n323 = local read "Invert APD Gate"() -> (w593:bool)
            n324 = Not(x=w591) -> (.not. x?=w592:bool)
            n325 = Select(t=w592, s=w593, f=w591) -> (s? t:f=w590:bool)
          }
        }
      }
    }
    frame Enabled {
    }
  }
  n326 = disable-structure shown="Disabled" {
    disable-tunnel: w3 -> [w625 _]
    frame Disabled {
      n327 = while "APD 1 Counter" {
        tunnel: w625 -> [_]
        stop <- FALSE stop-if-true
        n328 = flat-sequence {
          frame #0 {
            n329 = xnode "FPGA I/O Method Node"("FPGA I/O In"=refnum<k21> "Connector0/DIO0" ("APD 1 DO"), "Timeout"=-1) -> ()  [unwired: 2 out]
          }
          frame #1 {
            n330 = local read "APD1 int gate"() -> (w629:bool)
            n331 = case shown="True" w629 {
              frame False {
              }
              frame True {
                n332 = local read "APD1 out state"() -> (w630:bool)
                n333 = case shown="True" w630 {
                  frame False {
                    n334 = local read "APD 1 Counts 0"() -> (w632:u32)
                    n335 = Increment(x=w632) -> (x+1=→"APD 1 Counts 0":u32)
                  }
                  frame True {
                    n336 = local read "APD 1 Counts 1"() -> (w634:u32)
                    n337 = Increment(x=w634) -> (x+1=→"APD 1 Counts 1":u32)
                  }
                }
              }
            }
          }
        }
      }
      n338 = while "APD 2 Counter" {
        tunnel: w625 -> [_]
        stop <- FALSE stop-if-true
        n339 = flat-sequence {
          frame #0 {
            n340 = xnode "FPGA I/O Method Node"("FPGA I/O In"=refnum<k21> "Connector0/DIO1" ("APD 2 DO"), "Timeout"=-1) -> ()  [unwired: 2 out]
          }
          frame #1 {
            n341 = local read "APD2 int gate"() -> (w638:bool)
            n342 = case shown="True" w638 {
              frame False {
              }
              frame True {
                n343 = local read "APD2 out state"() -> (w639:bool)
                n344 = case shown="False" w639 {
                  frame False {
                    n345 = local read "APD 2 Counts 0"() -> (w641:u32)
                    n346 = Increment(x=w641) -> (x+1=→"APD 2 Counts 0":u32)
                  }
                  frame True {
                    n347 = local read "APD 2 Counts 1"() -> (w643:u32)
                    n348 = Increment(x=w643) -> (x+1=→"APD 2 Counts 1":u32)
                  }
                }
              }
            }
          }
        }
      }
    }
    frame Enabled {
    }
  }
  n349 = disable-structure shown="Disabled" {
    disable-tunnel: w7 -> [w645 _]
    disable-tunnel: w3 -> [w644 _]
    frame Disabled {
      n350 = while "APD 1 Gating" {
        shift-right: [w649] -> _
        shift-left: w644 -> [w654]
        shift-right: [w648] -> _
        shift-left: w645 -> [w646]
        stop <- FALSE stop-if-true
        n351 = flat-sequence {
          tunnel: w654 -> [w657]
          tunnel: [w658] -> w652
          tunnel: [w657] -> w650
          tunnel: [w656] -> w647
          tunnel: w646 -> [w656]
          tunnel: [w661] -> w653
          tunnel: w652 -> [w661]
          tunnel: [w660] -> w651
          tunnel: w650 -> [w660]
          tunnel: w647 -> [w659]
          tunnel: [w679] -> w649
          tunnel: w653 -> [w693]
          tunnel: w651 -> [w690]
          tunnel: [w662] -> w648
          frame #0 {
            n352 = call "Loop Timer7"("Count(Ticks)"=w657) -> ("Tick Count(Ticks)"=w658:u16)
          }
          frame #1 {
            # "Signal maybe then sent through \na transistor before APD"
            n353 = xnode "FPGA I/O Node"("Connector0/DIO4"=w659, "Connector0/DIO5"=w659, "Connector0/DIO6"=w659, "Connector0/DIO7"=w659) -> ()  [unwired: 4 in, 4 out]
            "APD1 int gate" <- w659
          }
          frame #2 {
            n354 = feedback #23(TRUE) -> (w685:bool)
            n355 = feedback-in #24(w693) -> ()
            n356 = feedback #24(w693) -> (w692:u16)
            n357 = Not(x=w685) -> (.not. x?=w682:bool)
            n358 = feedback-in #23(w682) -> ()
            n359 = Subtract(x=w693, y=w692) -> (x-y=w691:u16)
            n360 = Select(t="APD Gate ON Count", s=w682, f="APD Gate OFF Count") -> (s? t:f=w687:u16)
            n361 = Subtract(x=w691, y=w690) -> (x-y=w667:u16)
            n362 = Subtract(x=w687, y=w667) -> (x-y=w678:u16)
            n363 = Number To Boolean Array(number=w667) -> (Boolean array=w668:bool[])
            n364 = Or Array Elements(Boolean array=w668) -> (logical OR=w666:bool)
            n365 = Boolean To (0,1)(Boolean="+ phase (APD 1 Gate)") -> (0, 1=w676:i16)
            n366 = Boolean To (0,1)(Boolean=w666) -> (0, 1=w673:i16)
            n367 = Multiply(x=w676, y="Phase count adjustment (APD 1 Gate)") -> (x*y=w674:i16)
            n368 = To Unsigned Byte Integer(number=w673) -> (unsigned 8bit integer=w670:u8)
            n369 = Add(x=w678, y=w674) -> (x+y=w679:u16)
            n370 = feedback #25(i16 0) -> (w681:i16)
            n371 = Subtract(x=w681, y=w674) -> (x-y=w680:i16)
            "APD 1 Gate Relative Phase" <- w680
            n372 = feedback-in #25(w680) -> ()
            n373 = feedback #26(u8 0) -> (w671:u8)
            n374 = Add(x=w670, y=w671) -> (x+y=w669:u8)
            "APD 1 Gate Late Counter" <- w669
            n375 = feedback-in #26(w669) -> ()
            n376 = case shown="2" "APD Gate Operating Mode" {
              tunnel: [TRUE FALSE w696] -> w663
              tunnel: w685 -> [_ _ w696]
              frame 0, Default {
              }
              frame 1 {
              }
              frame 2 {
              }
            }
            n377 = Not(x=w663) -> (.not. x?=w664:bool)
            n378 = Select(t=w664, s="Invert APD Gate", f=w663) -> (s? t:f=w662:bool)
          }
        }
      }
    }
    frame Enabled {
    }
  }
  n379 = disable-structure shown="Disabled" {
    disable-tunnel: u16 0 -> [w699 _]
    disable-tunnel: w5 -> [w698 _]
    disable-tunnel: w3 -> [w697 _]
    frame Disabled {
      n380 = while "532 nm green fluorescent laser interlacing (DO to IA 532 nm AOM ME amp)." {
        shift-right: [w814] -> _
        shift-left: w697 -> [w819]
        shift-right: [w813] -> _
        shift-left: w698 -> [w811]
        stop <- FALSE stop-if-true
        n381 = flat-sequence {
          tunnel: w819 -> [w822]
          tunnel: [w823] -> w817
          tunnel: [w822] -> w815
          tunnel: [w821] -> w812
          tunnel: w811 -> [w821]
          tunnel: [w826] -> w818
          tunnel: w817 -> [w826]
          tunnel: [w825] -> w816
          tunnel: w815 -> [w825]
          tunnel: w812 -> [w824]
          tunnel: [w835] -> w814
          tunnel: w818 -> [w855]
          tunnel: w816 -> [w852]
          tunnel: [w844] -> w813
          frame #0 {
            n382 = call "Loop Timer4"("Count(Ticks)"=w822) -> ("Tick Count(Ticks)"=w823:u16)
          }
          frame #1 {
            n383 = xnode "FPGA I/O Node"("Connector1/DIO34"=w824, "Connector1/DIO38"=w824, "Connector1/DIO39"=w824) -> ()  [unwired: 3 in, 3 out]
          }
          frame #2 {
            n384 = feedback-in #27(w855) -> ()
            n385 = feedback #27(w855) -> (w854:u16)
            n386 = Subtract(x=w855, y=w854) -> (x-y=w853:u16)
            n387 = Subtract(x=w853, y=w852) -> (x-y=w828:u16)
            n388 = Number To Boolean Array(number=w828) -> (Boolean array=w829:bool[])
            n389 = Or Array Elements(Boolean array=w829) -> (logical OR=w827:bool)
            n390 = Boolean To (0,1)(Boolean="+ phase (GI)") -> (0, 1=w840:i16)
            n391 = Multiply(x=w840, y="Phase count adjustment (GI)") -> (x*y=w837:i16)
            n392 = Boolean To (0,1)(Boolean=w827) -> (0, 1=w834:i16)
            n393 = To Unsigned Byte Integer(number=w834) -> (unsigned 8bit integer=w831:u8)
            n394 = feedback #28(i16 0) -> (w838:i16)
            n395 = feedback #29(u8 0) -> (w832:u8)
            n396 = Add(x=w831, y=w832) -> (x+y=w830:u8)
            "GI Late Counter" <- w830
            n397 = feedback-in #29(w830) -> ()
            n398 = Subtract(x=w838, y=w837) -> (x-y=w836:i16)
            "GI Relative phase" <- w836
            n399 = feedback-in #28(w836) -> ()
            n400 = feedback #30(TRUE) -> (w847:bool)
            n401 = case shown="2" "Operating Mode" {
              tunnel: [TRUE FALSE w861] -> w844
              tunnel: w847 -> [_ _ w858]
              frame 0, Default {
              }
              frame 1 {
              }
              frame 2 {
                n402 = Not(x=w858) -> (.not. x?=w860:bool)
                n403 = Select(t=w860, s="Invert GI", f=w858) -> (s? t:f=w861:bool)
              }
            }
            n404 = Not(x=w847) -> (.not. x?=w843:bool)
            n405 = Select(t="Green interlace ON count", s=w843, f="Green interlace OFF count") -> (s? t:f=w849:u16)
            n406 = Subtract(x=w849, y=w828) -> (x-y=w841:u16)
            n407 = Add(x=w841, y=w837) -> (x+y=w835:u16)
            n408 = feedback-in #30(w843) -> ()
          }
        }
      }
      n409 = while "Green and red fluorescent laser interlacing (Current AO to IA 532 nm AOM ME amp)." {
        shift-right: [w708] -> _
        shift-left: w697 -> [w711]
        shift-right: [w705] -> _
        shift-left: w699 -> [w703]
        shift-right: [w702] -> _
        shift-left: w699 -> [w701]
        stop <- FALSE stop-if-true
        n410 = flat-sequence {
          tunnel: w711 -> [w715]
          tunnel: [w716] -> w710
          tunnel: [w715] -> w709
          tunnel: [w714] -> w704
          tunnel: w703 -> [w714]
          tunnel: w701 -> [w713]
          tunnel: [w713] -> w700
          tunnel: [w720] -> w707
          tunnel: w710 -> [w720]
          tunnel: [w719] -> w706
          tunnel: w709 -> [w719]
          tunnel: w704 -> [w718]
          tunnel: w700 -> [w717]
          tunnel: [w733] -> w708
          tunnel: [w749] -> w705
          tunnel: w707 -> [w760]
          tunnel: w706 -> [w757]
          tunnel: [w723] -> w702
          frame #0 {
            n411 = call "Loop Timer10"("Count(Ticks)"=w715) -> ("Tick Count(Ticks)"=w716:u16)
          }
          frame #1 {
            n412 = xnode "FPGA I/O Node"("Chassis2/Mod1/AO0"=w718, "Chassis2/Mod1/AO1"=w717) -> ()  [unwired: 2 in, 2 out]
          }
          frame #2 {
            # "Design note:\n\nThese two laser controls are in the same loop\nbecause the expansion current AI cannot separately\ntime the outputs fast enough for us.  Apparently\nit is because of communication time between the\nexpansion card and the fpga.\n\nSo the two analog control signals have the same timing\nand profile, but independent amplitudes to independently\ncontrol the intensity and feedback for each laser."
            n413 = feedback #31(TRUE) -> (w721:bool)
            n414 = Not(x=w721) -> (.not. x?=w722:bool)
            n415 = feedback-in #31(w722) -> ()
            n416 = Subtract(x="Green interlace OFF count 2", y="Green int current ON count adj") -> (x-y=w742:u16)
            n417 = disable-structure shown="Disabled" {
              disable-tunnel: [w764 _] -> w723
              disable-tunnel: w721 -> [w761 _]
              frame Disabled {
                n418 = case shown="2" "RI Operating Mode 2" {
                  tunnel: [TRUE FALSE w776] -> w762
                  tunnel: w761 -> [_ _ w773]
                  frame 0, Default {
                  }
                  frame 1 {
                  }
                  frame 2 {
                    n419 = Not(x=w773) -> (.not. x?=w775:bool)
                    n420 = Select(t=w775, s="Invert RI 2", f=w773) -> (s? t:f=w776:bool)
                  }
                }
                n421 = And(x=w762, y="Red FB On/Off") -> (x .and. y?=w770:bool)
                n422 = case shown="True" w770 {
                  tunnel: "RI Current Out" -> [w777 _]
                  tunnel: [w777 w786] -> w766
                  frame False {
                  }
                  frame True {
                    n423 = local read "Red FB Intensity"() -> (w782:i16)
                    n424 = Bundle("P4"="P4", "I4"="I4", "D4"="D4") -> (w778:cluster{"P4":i16, "I4":i16, "D4":i16})  [unwired: 1 in]
                    n425 = call "Slower PID.vi"("process variable"=w782, "reset?"="Red FB Reset", "setpoint"="Red FB Setpoint", "PID gains (x 2^8)"=w778, "output range"=cluster{"output high":i16, "output low":i16} {"output high"=32767, "output low"=-32768} ("Green FB output range")) -> ("output"=w789:i16)  [unwired: 10 out]
                    n426 = To Long Integer(number=w789) -> (32bit integer=w783:i32)
                    n427 = Add(x=w783, y=32768) -> (x+y=w785:i32)
                    n428 = To Unsigned Word Integer(number=w785) -> (unsigned 16bit integer=w786:u16)
                  }
                }
                n429 = Boolean To (0,1)(Boolean=w762) -> (0, 1=w765:i16)
                n430 = To Unsigned Word Integer(number=w765) -> (unsigned 16bit integer=w767:u16)
                n431 = Multiply(x=w767, y=w766) -> (x*y=w764:u16)
              }
              frame Enabled {
              }
            }
            n432 = feedback-in #32(w760) -> ()
            n433 = feedback #32(w760) -> (w759:u16)
            n434 = Add(x="Green int current ON count adj", y="Green interlace ON count 2") -> (x+y=w743:u16)
            n435 = Subtract(x=w760, y=w759) -> (x-y=w758:u16)
            n436 = Select(t=w743, s=w722, f=w742) -> (s? t:f=w754:u16)
            n437 = Subtract(x=w758, y=w757) -> (x-y=w726:u16)
            n438 = Subtract(x=w754, y=w726) -> (x-y=w737:u16)
            n439 = case shown="2" "Operating Mode 2" {
              tunnel: [TRUE FALSE w810] -> w724
              tunnel: w721 -> [_ _ w807]
              frame 0, Default {
              }
              frame 1 {
              }
              frame 2 {
                n440 = Not(x=w807) -> (.not. x?=w809:bool)
                n441 = Select(t=w809, s="Invert GI 2", f=w807) -> (s? t:f=w810:bool)
              }
            }
            n442 = Number To Boolean Array(number=w726) -> (Boolean array=w727:bool[])
            n443 = Boolean To (0,1)(Boolean="+ phase (GI) 2") -> (0, 1=w739:i16)
            n444 = Or Array Elements(Boolean array=w727) -> (logical OR=w725:bool)
            n445 = Boolean To (0,1)(Boolean=w725) -> (0, 1=w732:i16)
            n446 = Multiply(x=w739, y="Phase count adjustment (GI) 2") -> (x*y=w735:i16)
            n447 = To Unsigned Byte Integer(number=w732) -> (unsigned 8bit integer=w728:u8)
            n448 = Add(x=w737, y=w735) -> (x+y=w733:u16)
            n449 = feedback #33(u8 0) -> (w730:u8)
            n450 = Add(x=w728, y=w730) -> (x+y=w729:u8)
            "GI Late Counter 2" <- w729
            n451 = feedback-in #33(w729) -> ()
            n452 = feedback #34(i16 0) -> (w736:i16)
            n453 = Subtract(x=w736, y=w735) -> (x-y=w734:i16)
            "GI Relative phase 2" <- w734
            n454 = feedback-in #34(w734) -> ()
            n455 = And(x=w724, y="Green FB On/Off") -> (x .and. y?=w744:bool)
            n456 = case shown="False" w744 {
              tunnel: "Current Out" -> [w791 _]
              tunnel: [w791 w800] -> w748
              frame False {
              }
              frame True {
                n457 = local read "Green FB Sum"() -> (w796:i16)
                n458 = Bundle("P3"="P3", "I3"="I3", "D3"="D3") -> (w792:cluster{"P3":i16, "I3":i16, "D3":i16})  [unwired: 1 in]
                n459 = call "Slower PID.vi"("process variable"=w796, "reset?"="Green FB Reset", "setpoint"="Green FB Setpoint", "PID gains (x 2^8)"=w792, "output range"=cluster{"output high":i16, "output low":i16} {"output high"=32767, "output low"=-32768} ("Green FB output range")) -> ("output"=w803:i16)  [unwired: 10 out]
                n460 = To Long Integer(number=w803) -> (32bit integer=w797:i32)
                n461 = Add(x=w797, y=32768) -> (x+y=w799:i32)
                n462 = To Unsigned Word Integer(number=w799) -> (unsigned 16bit integer=w800:u16)
              }
            }
            n463 = Boolean To (0,1)(Boolean=w724) -> (0, 1=w750:i16)
            n464 = To Unsigned Word Integer(number=w750) -> (unsigned 16bit integer=w747:u16)
            n465 = Multiply(x=w747, y=w748) -> (x*y=w749:u16)
          }
        }
      }
    }
    frame Enabled {
    }
  }
  n466 = while "MCL stage control" {
    shift-right: [w874] -> _
    shift-left: w3 -> [w877]
    shift-right: [w867] -> _
    shift-left: w12 -> [w864]
    shift-right: [w866] -> _
    shift-left: w11 -> [w862]
    stop <- FALSE stop-if-true
    n467 = flat-sequence {
      tunnel: w877 -> [w881]
      tunnel: [w882] -> w873
      tunnel: [w881] -> w871
      tunnel: [w880] -> w865
      tunnel: w864 -> [w880]
      tunnel: [w879] -> w863
      tunnel: w862 -> [w879]
      tunnel: w873 -> [w886]
      tunnel: [w886] -> w872
      tunnel: w871 -> [w885]
      tunnel: [w885] -> w870
      tunnel: w865 -> [w884]
      tunnel: w863 -> [w883]
      tunnel: w872 -> [w894]
      tunnel: w870 -> [w893]
      tunnel: [w894] -> w876
      tunnel: [w893] -> w875
      tunnel: [w892] -> w869
      tunnel: [w891] -> w868
      tunnel: [w966] -> w874
      tunnel: w876 -> [w973]
      tunnel: w875 -> [w970]
      tunnel: w869 -> [w968]
      tunnel: w868 -> [w967]
      tunnel: [w968] -> w867
      tunnel: [w967] -> w866
      frame #0 {
        n468 = call "Loop Timer5"("Count(Ticks)"=w881) -> ("Tick Count(Ticks)"=w882:u32)
      }
      frame #1 {
        n469 = xnode "FPGA I/O Node"("Connector0/AO1"=w884, "Connector0/AO2"=w883) -> ()  [unwired: 2 in, 2 out]
      }
      frame #2 {
        n470 = local read "Scanning MCL"() -> (w906:bool)
        n471 = Or(x=w906, y="Start scan (MCL)") -> (x .or. y?=w901:bool)
        n472 = Not(x="Abort scan (MCL)") -> (.not. x?=w899:bool)
        n473 = And(x=w899, y=w901) -> (x .and. y?=w898:bool)
        n474 = case "Raster scan" shown="False" w898 {
          tunnel: [w907 w950] -> w903
          tunnel: "Start scan (MCL)" -> [_ w935]
          tunnel: [w907 w911] -> w887
          frame False {
            w907 = i16 0
            n475 = local write "Scanning MCL"(FALSE ("scanning")) -> ()
          }
          frame True {
            w921 = i16 0
            w920 = u64 0
            # "scan incr."
            # "freq. incr. mult."
            # "count steps"
            # "count number of cycles"
            n476 = feedback #35(w920) -> (w947:u64)
            n477 = Select(t=w920, s=w935, f=w947) -> (s? t:f=w949:u64)
            n478 = Increment(x=w949) -> (x+1=w946:u64)
            n479 = Greater?(x="Cycles per step (MCL)", y=w946) -> (0:w930:bool)
            n480 = Select(t=w946, s=w930, f=w920) -> (s? t:f=w945:u64)
            n481 = feedback-in #35(w945) -> ()
            n482 = feedback #36(w920) -> (w944:u64)
            n483 = Select(t=w920, s=w935, f=w944) -> (s? t:f=w939:u64)
            n484 = Increment(x=w939) -> (x+1=w943:u64)
            n485 = Add(x="Scan steps (MCL)", y="Scan steps (MCL)") -> (x+y=w942:u64)
            n486 = Select(t=w939, s=w930, f=w943) -> (s? t:f=w925:u64)
            n487 = Greater?(x=w942, y=w925) -> (0:w924:bool)
            n488 = Select(t=w925, s=w924, f=w920) -> (s? t:f=w940:u64)
            n489 = feedback-in #36(w940) -> ()
            n490 = Equal?(x="Scan steps (MCL)", y=w925) -> (x = y?=w929:bool)
            n491 = Greater?(x="Scan steps (MCL)", y=w939) -> (0:w938:bool)
            n492 = feedback #37(w921) -> (w941:i16)
            n493 = Select(t=w921, s=w935, f=w941) -> (s? t:f=w927:i16)
            n494 = Increment(x=w927) -> (x+1=w937:i16)
            n495 = Decrement(x=w927) -> (x-1=w936:i16)
            n496 = Select(t=w937, s=w938, f=w936) -> (s? t:f=w928:i16)
            n497 = Select(t=w927, s=w929, f=w928) -> (s? t:f=w926:i16)
            n498 = Select(t=w927, s=w930, f=w926) -> (s? t:f=w922:i16)
            n499 = Select(t=w922, s=w924, f=w921) -> (s? t:f=w923:i16)
            n500 = feedback-in #37(w923) -> ()
            n501 = feedback #38(w920) -> (w934:u64)
            n502 = Select(t=w920, s=w935, f=w934) -> (s? t:f=w909:u64)
            n503 = Increment(x=w909) -> (x+1=w931:u64)
            n504 = Select(t=w909, s=w924, f=w931) -> (s? t:f=w910:u64)
            n505 = Greater?(x="Number of scans (MCL)", y=w910) -> (0:w917:bool)
            n506 = Multiply(x="Scan freq.  increment (MCL)", y=w927) -> (x*y=w950:i16)
            n507 = Select(t=TRUE, s="Cont. Scan (MCL)", f=w917) -> (s? t:f=w916:bool)
            "Scanning MCL" <- w916
            n508 = Select(t=w910, s=w916, f=w920) -> (s? t:f=w932:u64)
            n509 = feedback-in #38(w932) -> ()
            n510 = Increment(x=w910) -> (x+1=→"Scan I (MCL)":u64)
            n511 = To Word Integer(number=w909) -> (16bit integer=w912:i16)
            n512 = Multiply(x=w912, y="Scan freq.  increment (MCL)") -> (x*y=w911:i16)
          }
        }
        n513 = Select(t=w887, s="1D or 2D Scan?", f=i16 0) -> (s? t:f=w888:i16)
        n514 = Select(t=w888, s="MCL Scan Axis", f=w903) -> (s? t:f=w902:i16)
        n515 = Select(t=w903, s="MCL Scan Axis", f=w888) -> (s? t:f=w904:i16)
        n516 = Add(x=w902, y="AO2") -> (x+y=w891:i16)
        n517 = Add(x="AO1", y=w904) -> (x+y=w892:i16)
      }
      frame #3 {
        n518 = feedback-in #39(w973) -> ()
        n519 = feedback #39(w973) -> (w972:u32)
        n520 = Boolean To (0,1)(Boolean="+ phase (MCL)") -> (0, 1=w964:i16)
        n521 = Subtract(x=w973, y=w972) -> (x-y=w971:u32)
        n522 = Multiply(x=w964, y="Phase count adjustment (MCL)") -> (x*y=w960:i16)
        n523 = Subtract(x=w971, y=w970) -> (x-y=w952:u32)
        n524 = Subtract(x="MCL count", y=w952) -> (x-y=w962:u32)
        n525 = feedback #40(i16 0) -> (w961:i16)
        n526 = Subtract(x=w961, y=w960) -> (x-y=w959:i16)
        "MCL Relative Phase" <- w959
        n527 = feedback-in #40(w959) -> ()
        n528 = Number To Boolean Array(number=w952) -> (Boolean array=w953:bool[])
        n529 = Or Array Elements(Boolean array=w953) -> (logical OR=w951:bool)
        n530 = Boolean To (0,1)(Boolean=w951) -> (0, 1=w958:i16)
        n531 = Add(x=w962, y=w960) -> (x+y=w966:u32)
        n532 = To Unsigned Byte Integer(number=w958) -> (unsigned 8bit integer=w955:u8)
        n533 = feedback #41(u8 0) -> (w956:u8)
        n534 = Add(x=w955, y=w956) -> (x+y=w954:u8)
        "MCL Late Counter" <- w954
        n535 = feedback-in #41(w954) -> ()
      }
    }
  }
  n536 = while "Control APD data integration - stream to host" {
    shift-right: [w978] -> _
    shift-left: w8 -> [w983]
    stop <- FALSE stop-if-true
    n537 = flat-sequence {
      tunnel: w983 -> [w985]
      tunnel: [w986] -> w981
      tunnel: [w985] -> w979
      tunnel: [w996] -> w982
      tunnel: w981 -> [w996]
      tunnel: [w995] -> w980
      tunnel: w979 -> [w995]
      tunnel: [w994] -> w977
      tunnel: [w993] -> w976
      tunnel: [w987] -> w975
      tunnel: [w1038] -> w978
      tunnel: w982 -> [w1048]
      tunnel: w980 -> [w1045]
      tunnel: w977 -> [w1031]
      tunnel: w976 -> [w1030]
      tunnel: w975 -> [w1018]
      frame #0 {
        n538 = call "Loop Timer6"("Count(Ticks)"=w985) -> ("Tick Count(Ticks)"=w986:u32)
      }
      frame #1 {
        n539 = flat-sequence {
          tunnel: [w998] -> w992
          tunnel: w992 -> [w1001]
          tunnel: [w1005] -> w991
          tunnel: [w1004] -> w990
          tunnel: [w1001] -> w989
          tunnel: [w1000] -> w988
          tunnel: [w1012] -> w993
          tunnel: [w1013] -> w994
          tunnel: w991 -> [w1013]
          tunnel: w990 -> [w1012]
          tunnel: w989 -> [w1011]
          tunnel: w988 -> [w1010]
          tunnel: [w1010] -> w987
          frame #0 {
            # "use separate variable so each APD won't\nhave to wait to read"
            n540 = feedback #42(FALSE) -> (w997:bool)
            "APD1 out state" <- w997
            "APD2 out state" <- w997
            "APD3 out state" <- w997
            n541 = Not(x=w997) -> (.not. x?=w998:bool)
            n542 = feedback-in #42(w998) -> ()
          }
          frame #1 {
            n543 = local read "APD 3 Counts 1"() -> (w1003:u32)
            n544 = local read "APD 3 Counts 0"() -> (w1002:u32)
            n545 = local read "APD 1 Counts 1"() -> (w1009:u32)
            n546 = local read "APD 1 Counts 0"() -> (w1008:u32)
            n547 = local read "APD 2 Counts 1"() -> (w1007:u32)
            n548 = local read "APD 2 Counts 0"() -> (w1006:u32)
            n549 = Select(t=w1003, s=w1001, f=w1002) -> (s? t:f=w1000:u32)
            n550 = Select(t=w1009, s=w1001, f=w1008) -> (s? t:f=w1005:u32)
            n551 = Select(t=w1007, s=w1001, f=w1006) -> (s? t:f=w1004:u32)
          }
          frame #2 {
            n552 = case shown="False" w1011 {
              frame False {
                w1014 = u32 0 ("APD 1 Counts 0")
                n553 = local write "APD 1 Counts 0"(w1014) -> ()
                n554 = local write "APD 2 Counts 0"(w1014) -> ()
                n555 = local write "APD 3 Counts 0"(w1014) -> ()
              }
              frame True {
                w1015 = u32 0 ("APD 1 Counts 1")
                n556 = local write "APD 1 Counts 1"(w1015) -> ()
                n557 = local write "APD 2 Counts 1"(w1015) -> ()
                n558 = local write "APD 3 Counts 1"(w1015) -> ()
              }
            }
          }
        }
      }
      frame #2 {
        n559 = feedback-in #43(w1048) -> ()
        n560 = feedback #43(w1048) -> (w1047:u32)
        n561 = Subtract(x=w1048, y=w1047) -> (x-y=w1046:u32)
        n562 = Subtract(x=w1046, y=w1045) -> (x-y=w1023:u32)
        n563 = case shown="True" "APD to FIFO" {
          tunnel: w1031 -> [_ w1053]
          tunnel: w1030 -> [_ w1051]
          tunnel: w1018 -> [_ w1049]
          frame False {
          }
          frame True {
            n564 = flat-sequence {
              tunnel: 0 ("Timeout") -> [w1055]
              tunnel: w1053 -> [w1056]
              tunnel: [w1055] -> w1052
              tunnel: w1052 -> [w1057]
              tunnel: w1051 -> [w1058]
              tunnel: [w1057] -> w1050
              tunnel: w1050 -> [w1060]
              tunnel: w1049 -> [w1059]
              frame #0 {
                n565 = xnode ("FIFO Write")("Element"=w1056, "Timeout"=w1055) -> ()  [unwired: 1 in, 2 out]
              }
              frame #1 {
                n566 = xnode ("FIFO Write")("Element"=w1058, "Timeout"=w1057) -> ()  [unwired: 1 in, 2 out]
              }
              frame #2 {
                n567 = xnode ("FIFO Write")("Element"=w1059, "Timeout"=w1060) -> ()  [unwired: 1 in, 2 out]
              }
            }
          }
        }
        n568 = Subtract(x="APD Acq Rate Count", y=w1023) -> (x-y=w1039:u32)
        n569 = Number To Boolean Array(number=w1023) -> (Boolean array=w1024:bool[])
        n570 = Or Array Elements(Boolean array=w1024) -> (logical OR=w1022:bool)
        n571 = Boolean To (0,1)(Boolean=w1022) -> (0, 1=w1029:i16)
        n572 = To Unsigned Byte Integer(number=w1029) -> (unsigned 8bit integer=w1026:u8)
        n573 = feedback #44(u8 0) -> (w1027:u8)
        n574 = Add(x=w1026, y=w1027) -> (x+y=w1025:u8)
        "APD Acq Late Counter" <- w1025
        n575 = feedback-in #44(w1025) -> ()
        n576 = Boolean To (0,1)(Boolean="+ phase (APD Acq)") -> (0, 1=w1035:i16)
        n577 = Multiply(x=w1035, y="Phase Count Adjustment (APD Acq)") -> (x*y=w1032:i16)
        n578 = Add(x=w1039, y=w1032) -> (x+y=w1038:u32)
        n579 = feedback #45(i16 0) -> (w1037:i16)
        n580 = Subtract(x=w1037, y=w1032) -> (x-y=w1034:i16)
        "APD Acq Relative Phase" <- w1034
        n581 = feedback-in #45(w1034) -> ()
        n582 = To Word Integer(number=w1031) -> (16bit integer=w1040:i16)
        n583 = To Word Integer(number=w1018) -> (16bit integer=w1019:i16)
        n584 = To Word Integer(number=w1030) -> (16bit integer=w1041:i16)
        n585 = Multiply(x="APD AO scale factor", y=w1041) -> (x*y=w1020:i16)
        n586 = Multiply(x="APD AO scale factor", y=w1019) -> (x*y=w1016:i16)
        n587 = Multiply(x="APD AO scale factor", y=w1040) -> (x*y=w1021:i16)
        n588 = xnode "FPGA I/O Node"("Connector0/AO6"=w1021, "Connector0/AO7"=w1020, "Connector0/AO5"=w1016) -> ()  [unwired: 3 in, 3 out]
      }
    }
  }
  n589 = while "DAQ AI set 1" {
    shift-right: [w1061] -> _
    shift-left: w3 -> [w1066]
    stop <- FALSE stop-if-true
    n590 = flat-sequence {
      tunnel: w1066 -> [w1076]
      tunnel: [w1077] -> w1064
      tunnel: [w1076] -> w1063
      tunnel: [w1087] -> w1074
      tunnel: [w1086] -> w1073
      tunnel: [w1085] -> w1072
      tunnel: [w1084] -> w1071
      tunnel: [w1083] -> w1070
      tunnel: [w1082] -> w1069
      tunnel: [w1081] -> w1068
      tunnel: [w1080] -> w1067
      tunnel: [w1079] -> w1065
      tunnel: w1064 -> [w1079]
      tunnel: w1063 -> [w1078]
      tunnel: [w1078] -> w1062
      tunnel: [w1119] -> w1061
      tunnel: w1074 -> [w1145]
      tunnel: w1073 -> [w1111]
      tunnel: w1072 -> [w1112]
      tunnel: w1071 -> [w1092]
      tunnel: w1070 -> [w1135]
      tunnel: w1069 -> [w1134]
      tunnel: w1068 -> [w1133]
      tunnel: w1067 -> [w1132]
      tunnel: w1065 -> [w1129]
      tunnel: w1062 -> [w1126]
      frame #0 {
        n591 = call "Loop Timer3"("Count(Ticks)"=w1076) -> ("Tick Count(Ticks)"=w1077:u16)
      }
      frame #1 {
        n592 = xnode "FPGA I/O Node"("Connector1/DIO31"=TRUE ("Connector1/DIO33")) -> ("Connector0/AI0"=w1087:i16, "Connector0/AI1"=w1086:i16, "Connector0/AI2"=w1085:i16, "Connector0/AI3"=w1084:i16, "Connector0/AI4"=w1083:i16, "Connector0/AI5"=w1082:i16, "Connector0/AI6"=w1081:i16, "Connector0/AI7"=w1080:i16)  [unwired: 9 in, 9 out]
      }
      frame #2 {
        w1115 = FALSE ("AI to FIFO")
        # "Changed by Ronen - the X and Y values of the MCL trap are now sent to the trap position FIFO"
        # "Adjust phase after data acquired if button pressed"
        n593 = feedback #46(i16 1) -> (w1138:i16)
        n594 = Increment(x=w1138) -> (x+1=w1144:i16)
        n595 = Scale By Power Of 2(n="AI1 X Scale", x=w1111) -> (x*2^n=w1109:i16)
        n596 = Greater?(x=w1144, y="N of AI1 Int Acq Sets") -> (0:w1141:bool)
        n597 = Select(t=i16 1, s=w1141, f=w1144) -> (s? t:f=w1143:i16)
        n598 = feedback-in #46(w1143) -> ()
        n599 = Divide(x=w1109, y=w1092) -> (x/y=w1108:fxp<+/-,16,1>)
        n600 = feedback #47(w1115) -> (w1113:bool)
        n601 = feedback #48(w1115) -> (w1131:bool)
        n602 = case shown="1, Default" w1138 {
          tunnel: w1112 -> [w1170 w1177 _]
          tunnel: ["Set 1" "Set 2" "Set 3"] -> w1136
          tunnel: ["AI to FIFO" w1179 w1184] -> w1130
          tunnel: w1131 -> [_ w1179 w1184]
          tunnel: ["Trap Pos to FIFO" w1178 w1183] -> w1114
          tunnel: w1113 -> [_ w1178 w1183]
          tunnel: w1108 -> [w1169 w1176 _]
          tunnel: [w1168 w1174 FALSE] -> w1091
          tunnel: [w1167 w1175 u64 0 ("BD1 Frequency Out 2")] -> w1095
          frame 1, Default {
            n603 = local read "BD1 Frequency Out 1"() -> (w1167:u64)
            n604 = Compound Arithmetic op=AND("Trap Pos to FIFO", "Set 1", "AI to FIFO") -> (w1168:bool)
            "AI2 Y Sum Set 1" <- w1170
            "AI1 X Set 1" <- w1169
          }
          frame 2 {
            n605 = local read "BD1 Frequency Out 2"() -> (w1175:u64)
            n606 = Compound Arithmetic op=AND(w1178, "Set 2", w1179) -> (w1174:bool)
            "AI2 Y Sum Set 2" <- w1177
            "AI1 X Set 2" <- w1176
          }
          frame 3 {
          }
        }
        n607 = And(x=w1136, y=w1130) -> (x .and. y?=w1137:bool)
        n608 = case shown="True" w1137 {
          tunnel: w1145 -> [_ w1198]
          tunnel: w1111 -> [_ w1197]
          tunnel: w1112 -> [_ w1196]
          tunnel: w1092 -> [_ w1195]
          tunnel: w1135 -> [_ w1194]
          tunnel: w1134 -> [_ w1193]
          tunnel: w1133 -> [_ w1192]
          tunnel: w1132 -> [_ w1191]
          tunnel: 0 ("DMA buffer timeout") -> [_ w1200]
          frame False {
          }
          frame True {
            n609 = Build Array(w1198, w1197, w1196, w1195, w1194, w1193, w1192, w1191) -> (w1199:i16[])
            n610 = for {
              tunnel: w1199 -> [w1202] mode=indexing
              tunnel: w1200 -> [w1203]
              tunnel: [w1201] -> w1189 mode=indexing
              n611 = xnode ("FIFO Write")("Element"=w1202, "Timeout"=w1203) -> ("Timed Out?"=w1201:bool)  [unwired: 1 in, 1 out]
            }
            n612 = Or Array Elements(Boolean array=w1189) -> (logical OR=w1186:bool)
            n613 = Boolean To (0,1)(Boolean=w1186) -> (0, 1=w1188:i16)
            n614 = feedback #49(u16 0) -> (w1187:u16)
            n615 = Add(x=w1188, y=w1187) -> (x+y=w1185:u16)
            "Trap AI FIFO Timeout" <- w1185
            n616 = feedback-in #49(w1185) -> ()
          }
        }
        n617 = feedback-in #47(w1114) -> ()
        n618 = feedback-in #48(w1130) -> ()
        n619 = local read "Piezo Y out"() -> (w1089:u16)
        n620 = local read "Piezo X out"() -> (w1090:u16)
        n621 = case shown="True" w1091 {
          tunnel: w1095 -> [_ w1153]
          tunnel: [u8 0 w1150] -> w1094
          tunnel: w1090 -> [_ w1149]
          tunnel: w1089 -> [_ w1148]
          frame False {
          }
          frame True {
            n622 = Split Number(x=w1153) -> (hi(x)=w1154:u32, lo(x)=w1155:u32)
            n623 = Split Number(x=w1154) -> (lo(x)=w1156:u16)  [unwired: 1 out]
            n624 = Split Number(x=w1155) -> (hi(x)=w1157:u16, lo(x)=w1158:u16)
            n625 = Build Array "BD 1 nu Stack"(w1156, w1157, w1158, w1149, w1148) -> (w1152:u16[])
            n626 = for {
              tunnel: w1152 -> [w1165] mode=indexing
              shift-right: [w1161] -> w1150
              shift-left: u8 0 -> [w1162]
              n627 = xnode ("FIFO Method Node")("Element"=w1165, "Timeout"="Trap FIFO Set Timeout") -> ("Timed Out?"=w1164:bool)  [unwired: 1 in, 1 out]
              n628 = Boolean To (0,1)(Boolean=w1164) -> (0, 1=w1163:i16)
              n629 = To Unsigned Byte Integer(number=w1163) -> (unsigned 8bit integer=w1160:u8)
              n630 = Add(x=w1160, y=w1162) -> (x+y=w1161:u8)
            }
          }
        }
        n631 = To Unsigned Word Integer(number=w1094) -> (unsigned 16bit integer=w1093:u16)
        n632 = feedback #50(u16 0) -> (w1106:u16)
        n633 = Add(x=w1093, y=w1106) -> (x+y=w1105:u16)
        "Trap Pos FIFO Timeout" <- w1105
        n634 = feedback-in #50(w1105) -> ()
        n635 = feedback-in #51(w1129) -> ()
        n636 = feedback #51(w1129) -> (w1128:u16)
        n637 = Subtract(x=w1129, y=w1128) -> (x-y=w1127:u16)
        n638 = xnode "FPGA I/O Node"("Connector1/DIO31"=FALSE ("Connector1/DIO34")) -> ()  [unwired: 1 in, 1 out]
        n639 = Subtract(x=w1127, y=w1126) -> (x-y=w1097:u16)
        n640 = Boolean To (0,1)(Boolean="+ phase") -> (0, 1=w1122:i16)
        n641 = Multiply(x=w1122, y="Phase count adjustment") -> (x*y=w1116:i16)
        n642 = Subtract(x="ai count", y=w1097) -> (x-y=w1120:u16)
        n643 = Number To Boolean Array(number=w1097) -> (Boolean array=w1098:bool[])
        n644 = feedback #52(i16 0) -> (w1118:i16)
        n645 = Add(x=w1120, y=w1116) -> (x+y=w1119:u16)
        n646 = Subtract(x=w1118, y=w1116) -> (x-y=w1117:i16)
        "Relative phase" <- w1117
        n647 = feedback-in #52(w1117) -> ()
        n648 = Or Array Elements(Boolean array=w1098) -> (logical OR=w1096:bool)
        n649 = Boolean To (0,1)(Boolean=w1096) -> (0, 1=w1103:i16)
        n650 = To Unsigned Byte Integer(number=w1103) -> (unsigned 8bit integer=w1100:u8)
        n651 = feedback #53(u8 0) -> (w1101:u8)
        n652 = Add(x=w1100, y=w1101) -> (x+y=w1099:u8)
        "AI Late Counter" <- w1099
        n653 = feedback-in #53(w1099) -> ()
      }
    }
  }
  n654 = node-c288(w9) -> ()
  n655 = disable-structure shown="Disabled" {
    disable-tunnel: w3 -> [w1204 _]
    frame Disabled {
      n656 = while "APD 3 Counter" {
        tunnel: w1204 -> [_]
        stop <- FALSE stop-if-true
        n657 = flat-sequence {
          frame #0 {
            n658 = xnode "FPGA I/O Method Node"("FPGA I/O In"=refnum<k21> "Connector0/DIO2" ("APD 2 DO"), "Timeout"=-1) -> ()  [unwired: 2 out]
          }
          frame #1 {
            n659 = local read "APD3 int gate"() -> (w1208:bool)
            n660 = case shown="True" w1208 {
              frame False {
              }
              frame True {
                n661 = local read "APD3 out state"() -> (w1209:bool)
                n662 = case shown="True" w1209 {
                  frame False {
                    n663 = local read "APD 3 Counts 0"() -> (w1211:u32)
                    n664 = Increment(x=w1211) -> (x+1=→"APD 3 Counts 0":u32)
                  }
                  frame True {
                    n665 = local read "APD 3 Counts 1"() -> (w1213:u32)
                    n666 = Increment(x=w1213) -> (x+1=→"APD 3 Counts 1":u32)
                  }
                }
              }
            }
          }
        }
      }
    }
    frame Enabled {
    }
  }
  n667 = disable-structure shown="Disabled" {
    disable-tunnel: w7 -> [w1215 _]
    disable-tunnel: w3 -> [w1214 _]
    frame Disabled {
      n668 = while "APD 3 Gating" {
        shift-right: [w1219] -> _
        shift-left: w1214 -> [w1224]
        shift-right: [w1218] -> _
        shift-left: w1215 -> [w1216]
        stop <- FALSE stop-if-true
        n669 = flat-sequence {
          tunnel: w1224 -> [w1227]
          tunnel: [w1228] -> w1222
          tunnel: [w1227] -> w1220
          tunnel: [w1226] -> w1217
          tunnel: w1216 -> [w1226]
          tunnel: [w1231] -> w1223
          tunnel: w1222 -> [w1231]
          tunnel: [w1230] -> w1221
          tunnel: w1220 -> [w1230]
          tunnel: w1217 -> [w1229]
          tunnel: [w1252] -> w1219
          tunnel: w1223 -> [w1263]
          tunnel: w1221 -> [w1260]
          tunnel: [w1232] -> w1218
          frame #0 {
            n670 = call "Loop Timer15"("Count(Ticks)"=w1227) -> ("Tick Count(Ticks)"=w1228:u16)
          }
          frame #1 {
            # "Signal maybe then sent through \na transistor before APD"
            n671 = xnode "FPGA I/O Node"("Connector0/DIO12"=w1229, "Connector0/DIO13"=w1229, "Connector0/DIO14"=w1229, "Connector0/DIO15"=w1229) -> ()  [unwired: 4 in, 4 out]
            "APD3 int gate" <- w1229
          }
          frame #2 {
            n672 = local read "APD Gate OFF Count"() -> (w1237:u16)
            n673 = local read "APD Gate ON Count"() -> (w1238:u16)
            n674 = feedback #54(TRUE) -> (w1257:bool)
            n675 = feedback-in #55(w1263) -> ()
            n676 = feedback #55(w1263) -> (w1262:u16)
            n677 = Not(x=w1257) -> (.not. x?=w1255:bool)
            n678 = feedback-in #54(w1255) -> ()
            n679 = Subtract(x=w1263, y=w1262) -> (x-y=w1261:u16)
            n680 = Select(t=w1238, s=w1255, f=w1237) -> (s? t:f=w1259:u16)
            n681 = Subtract(x=w1261, y=w1260) -> (x-y=w1240:u16)
            n682 = Subtract(x=w1259, y=w1240) -> (x-y=w1251:u16)
            n683 = Number To Boolean Array(number=w1240) -> (Boolean array=w1241:bool[])
            n684 = Or Array Elements(Boolean array=w1241) -> (logical OR=w1239:bool)
            n685 = Boolean To (0,1)(Boolean=w1239) -> (0, 1=w1246:i16)
            n686 = Boolean To (0,1)(Boolean="+ phase (APD 3 Gate)") -> (0, 1=w1249:i16)
            n687 = To Unsigned Byte Integer(number=w1246) -> (unsigned 8bit integer=w1243:u8)
            n688 = Multiply(x=w1249, y="Phase count adjustment (APD 3 Gate)") -> (x*y=w1247:i16)
            n689 = feedback #56(u8 0) -> (w1244:u8)
            n690 = Add(x=w1243, y=w1244) -> (x+y=w1242:u8)
            "APD 3 Gate Late Counter" <- w1242
            n691 = feedback-in #56(w1242) -> ()
            n692 = Add(x=w1251, y=w1247) -> (x+y=w1252:u16)
            n693 = feedback #57(i16 0) -> (w1254:i16)
            n694 = Subtract(x=w1254, y=w1247) -> (x-y=w1253:i16)
            "APD 3 Gate Relative Phase" <- w1253
            n695 = feedback-in #57(w1253) -> ()
            n696 = local read "APD Gate Operating Mode"() -> (w1236:u8)
            n697 = case shown="2" w1236 {
              tunnel: [TRUE FALSE w1266] -> w1233
              tunnel: w1257 -> [_ _ w1266]
              frame 0, Default {
              }
              frame 1 {
              }
              frame 2 {
              }
            }
            n698 = local read "Invert APD Gate"() -> (w1235:bool)
            n699 = Not(x=w1233) -> (.not. x?=w1234:bool)
            n700 = Select(t=w1234, s=w1235, f=w1233) -> (s? t:f=w1232:bool)
          }
        }
      }
    }
    frame Enabled {
    }
  }
  n701 = disable-structure shown="Disabled" {
    disable-tunnel: w5 -> [w1268 _]
    disable-tunnel: w3 -> [w1267 _]
    frame Disabled {
      n702 = while "633 nm red  fluorescent laser interlacing (DO to IA 633 nm AOM ME amp)." {
        shift-right: [w1272] -> _
        shift-left: w1267 -> [w1277]
        shift-right: [w1271] -> _
        shift-left: w1268 -> [w1269]
        stop <- FALSE stop-if-true
        n703 = flat-sequence {
          tunnel: w1277 -> [w1280]
          tunnel: [w1281] -> w1275
          tunnel: [w1280] -> w1273
          tunnel: [w1279] -> w1270
          tunnel: w1269 -> [w1279]
          tunnel: [w1284] -> w1276
          tunnel: w1275 -> [w1284]
          tunnel: [w1283] -> w1274
          tunnel: w1273 -> [w1283]
          tunnel: w1270 -> [w1282]
          tunnel: [w1293] -> w1272
          tunnel: w1276 -> [w1313]
          tunnel: w1274 -> [w1310]
          tunnel: [w1302] -> w1271
          frame #0 {
            n704 = call "Loop Timer11"("Count(Ticks)"=w1280) -> ("Tick Count(Ticks)"=w1281:u16)
          }
          frame #1 {
            # "Then to PRL 440 amp"
            n705 = xnode "FPGA I/O Node"("Connector1/DIO32"=w1282) -> ()  [unwired: 1 in, 1 out]
          }
          frame #2 {
            n706 = feedback-in #58(w1313) -> ()
            n707 = feedback #58(w1313) -> (w1312:u16)
            n708 = Subtract(x=w1313, y=w1312) -> (x-y=w1311:u16)
            n709 = Subtract(x=w1311, y=w1310) -> (x-y=w1286:u16)
            n710 = Number To Boolean Array(number=w1286) -> (Boolean array=w1287:bool[])
            n711 = Or Array Elements(Boolean array=w1287) -> (logical OR=w1285:bool)
            n712 = Boolean To (0,1)(Boolean="+ phase (RI)") -> (0, 1=w1298:i16)
            n713 = Multiply(x=w1298, y="Phase count adjustment (RI)") -> (x*y=w1295:i16)
            n714 = Boolean To (0,1)(Boolean=w1285) -> (0, 1=w1292:i16)
            n715 = To Unsigned Byte Integer(number=w1292) -> (unsigned 8bit integer=w1289:u8)
            n716 = feedback #59(i16 0) -> (w1296:i16)
            n717 = feedback #60(u8 0) -> (w1290:u8)
            n718 = Add(x=w1289, y=w1290) -> (x+y=w1288:u8)
            "RI Late Counter" <- w1288
            n719 = feedback-in #60(w1288) -> ()
            n720 = Subtract(x=w1296, y=w1295) -> (x-y=w1294:i16)
            "RI Relative phase" <- w1294
            n721 = feedback-in #59(w1294) -> ()
            n722 = feedback #61(TRUE) -> (w1305:bool)
            n723 = case shown="2" "Red Laser Operating Mode" {
              tunnel: [TRUE FALSE w1319] -> w1302
              tunnel: w1305 -> [_ _ w1316]
              frame 0, Default {
              }
              frame 1 {
              }
              frame 2 {
                n724 = Not(x=w1316) -> (.not. x?=w1318:bool)
                n725 = Select(t=w1318, s="Invert RI", f=w1316) -> (s? t:f=w1319:bool)
              }
            }
            n726 = Not(x=w1305) -> (.not. x?=w1301:bool)
            n727 = Select(t="Red interlace ON count", s=w1301, f="Red interlace OFF count") -> (s? t:f=w1307:u16)
            n728 = Subtract(x=w1307, y=w1286) -> (x-y=w1299:u16)
            n729 = Add(x=w1299, y=w1295) -> (x+y=w1293:u16)
            n730 = feedback-in #61(w1301) -> ()
          }
        }
      }
    }
    frame Enabled {
    }
  }
  n731 = disable-structure shown="Disabled" {
    disable-tunnel: w3 -> [w1320 _]
    frame Disabled {
      n732 = while "Blue fluorescent laser interlacing (AO control direct to laser)." {
        shift-right: [w1327] -> _
        shift-left: w1320 -> [w1330]
        shift-right: [w1324] -> _
        shift-left: i16 0 -> [w1322]
        stop <- FALSE stop-if-true
        n733 = flat-sequence {
          tunnel: w1330 -> [w1333]
          tunnel: [w1334] -> w1329
          tunnel: [w1333] -> w1328
          tunnel: [w1332] -> w1323
          tunnel: w1322 -> [w1332]
          tunnel: [w1337] -> w1326
          tunnel: w1329 -> [w1337]
          tunnel: [w1336] -> w1325
          tunnel: w1328 -> [w1336]
          tunnel: w1323 -> [w1335]
          tunnel: [w1347] -> w1327
          tunnel: [w1363] -> w1324
          tunnel: w1326 -> [w1375]
          tunnel: w1325 -> [w1372]
          frame #0 {
            n734 = call "Loop Timer13"("Count(Ticks)"=w1333) -> ("Tick Count(Ticks)"=w1334:u16)
          }
          frame #1 {
            n735 = xnode "FPGA I/O Node"("Connector0/AO3"=w1335) -> ()  [unwired: 1 in, 1 out]
          }
          frame #2 {
            n736 = Subtract(x="Blue OFF count (AO)", y="Blue current ON count adj (AO)") -> (x-y=w1356:u16)
            n737 = feedback-in #62(w1375) -> ()
            n738 = feedback #62(w1375) -> (w1374:u16)
            n739 = Add(x="Blue current ON count adj (AO)", y="Blue ON count (AO)") -> (x+y=w1357:u16)
            n740 = Subtract(x=w1375, y=w1374) -> (x-y=w1373:u16)
            n741 = Subtract(x=w1373, y=w1372) -> (x-y=w1340:u16)
            n742 = Number To Boolean Array(number=w1340) -> (Boolean array=w1341:bool[])
            n743 = Boolean To (0,1)(Boolean="+ phase (BI AO)") -> (0, 1=w1353:i16)
            n744 = Or Array Elements(Boolean array=w1341) -> (logical OR=w1339:bool)
            n745 = Boolean To (0,1)(Boolean=w1339) -> (0, 1=w1346:i16)
            n746 = Multiply(x=w1353, y="Phase count adjustment (BI AO)") -> (x*y=w1349:i16)
            n747 = To Unsigned Byte Integer(number=w1346) -> (unsigned 8bit integer=w1342:u8)
            n748 = feedback #63(u8 0) -> (w1344:u8)
            n749 = Add(x=w1342, y=w1344) -> (x+y=w1343:u8)
            "BI Late Counter (AO)" <- w1343
            n750 = feedback-in #63(w1343) -> ()
            n751 = feedback #64(i16 0) -> (w1350:i16)
            n752 = Subtract(x=w1350, y=w1349) -> (x-y=w1348:i16)
            "BI Relative phase (AO)" <- w1348
            n753 = feedback-in #64(w1348) -> ()
            n754 = feedback #65(TRUE) -> (w1367:bool)
            n755 = case shown="2" "BI Operating Mode (AO)" {
              tunnel: [TRUE FALSE w1391] -> w1358
              tunnel: w1367 -> [_ _ w1388]
              frame 0, Default {
              }
              frame 1 {
              }
              frame 2 {
                n756 = Not(x=w1388) -> (.not. x?=w1390:bool)
                n757 = Select(t=w1390, s="Invert BI (AO)", f=w1388) -> (s? t:f=w1391:bool)
              }
            }
            n758 = And(x=w1358, y="Blue FB On/Off") -> (x .and. y?=w1359:bool)
            n759 = case shown="True" w1359 {
              tunnel: "BI Current Out" -> [w1376 _]
              tunnel: [w1376 w1378] -> w1362
              frame False {
              }
              frame True {
                n760 = local read "Blue Intensity"() -> (w1377:i16)
                n761 = Bundle("P5"="P5", "I5"="I5", "D5"="D5") -> (w1379:cluster{"P5":i16, "I5":i16, "D5":i16})  [unwired: 1 in]
                n762 = call "Slower PID.vi"("process variable"=w1377, "reset?"="Blue FB Reset", "setpoint"="Blue FB Setpoint", "PID gains (x 2^8)"=w1379, "output range"=cluster{"output high":i16, "output low":i16} {"output high"=32767, "output low"=0} ("Green FB output range")) -> ("output"=w1378:i16)  [unwired: 10 out]
              }
            }
            n763 = Not(x=w1367) -> (.not. x?=w1364:bool)
            n764 = Select(t=w1357, s=w1364, f=w1356) -> (s? t:f=w1369:u16)
            n765 = Subtract(x=w1369, y=w1340) -> (x-y=w1351:u16)
            n766 = Add(x=w1351, y=w1349) -> (x+y=w1347:u16)
            n767 = feedback-in #65(w1364) -> ()
            n768 = Boolean To (0,1)(Boolean=w1358) -> (0, 1=w1338:i16)
            n769 = Multiply(x=w1338, y=w1362) -> (x*y=w1363:i16)
          }
        }
      }
    }
    frame Enabled {
    }
  }
  n770 = disable-structure shown="Disabled" {
    disable-tunnel: w5 -> [w1393 _]
    disable-tunnel: w3 -> [w1392 _]
    frame Disabled {
      n771 = while "473 nm blue  fluorescent laser interlacing (DO to blue laser digital control input)." {
        shift-right: [w1397] -> _
        shift-left: w1392 -> [w1402]
        shift-right: [w1396] -> _
        shift-left: w1393 -> [w1394]
        stop <- FALSE stop-if-true
        n772 = flat-sequence {
          tunnel: w1402 -> [w1405]
          tunnel: [w1406] -> w1400
          tunnel: [w1405] -> w1398
          tunnel: [w1404] -> w1395
          tunnel: w1394 -> [w1404]
          tunnel: [w1409] -> w1401
          tunnel: w1400 -> [w1409]
          tunnel: [w1408] -> w1399
          tunnel: w1398 -> [w1408]
          tunnel: w1395 -> [w1407]
          tunnel: [w1418] -> w1397
          tunnel: w1401 -> [w1438]
          tunnel: w1399 -> [w1435]
          tunnel: [w1427] -> w1396
          frame #0 {
            n773 = call "Loop Timer14"("Count(Ticks)"=w1405) -> ("Tick Count(Ticks)"=w1406:u16)
          }
          frame #1 {
            n774 = xnode "FPGA I/O Node"("Connector1/DIO28"=w1407) -> ()  [unwired: 1 in, 1 out]
          }
          frame #2 {
            n775 = feedback-in #66(w1438) -> ()
            n776 = feedback #66(w1438) -> (w1437:u16)
            n777 = Subtract(x=w1438, y=w1437) -> (x-y=w1436:u16)
            n778 = Subtract(x=w1436, y=w1435) -> (x-y=w1411:u16)
            n779 = Number To Boolean Array(number=w1411) -> (Boolean array=w1412:bool[])
            n780 = Or Array Elements(Boolean array=w1412) -> (logical OR=w1410:bool)
            n781 = Boolean To (0,1)(Boolean="+ phase (BI D)") -> (0, 1=w1423:i16)
            n782 = Multiply(x=w1423, y="Phase count adjustment (BI D)") -> (x*y=w1420:i16)
            n783 = Boolean To (0,1)(Boolean=w1410) -> (0, 1=w1417:i16)
            n784 = To Unsigned Byte Integer(number=w1417) -> (unsigned 8bit integer=w1414:u8)
            n785 = feedback #67(i16 0) -> (w1421:i16)
            n786 = feedback #68(u8 0) -> (w1415:u8)
            n787 = Add(x=w1414, y=w1415) -> (x+y=w1413:u8)
            "Blue Late Counter (D)" <- w1413
            n788 = feedback-in #68(w1413) -> ()
            n789 = Subtract(x=w1421, y=w1420) -> (x-y=w1419:i16)
            "BI Relative phase (D)" <- w1419
            n790 = feedback-in #67(w1419) -> ()
            n791 = feedback #69(TRUE) -> (w1430:bool)
            n792 = case shown="2" "Blue Laser Operating Mode (D)" {
              tunnel: [TRUE FALSE w1444] -> w1427
              tunnel: w1430 -> [_ _ w1441]
              frame 0, Default {
              }
              frame 1 {
              }
              frame 2 {
                n793 = Not(x=w1441) -> (.not. x?=w1443:bool)
                n794 = Select(t=w1443, s="Invert BI (D)", f=w1441) -> (s? t:f=w1444:bool)
              }
            }
            n795 = Not(x=w1430) -> (.not. x?=w1426:bool)
            n796 = Select(t="Blue interlace ON count (D)", s=w1426, f="Blue interlace OFF count (D)") -> (s? t:f=w1432:u16)
            n797 = Subtract(x=w1432, y=w1411) -> (x-y=w1424:u16)
            n798 = Add(x=w1424, y=w1420) -> (x+y=w1418:u16)
            n799 = feedback-in #69(w1426) -> ()
          }
        }
      }
    }
    frame Enabled {
    }
  }
